vi "Interfaz grafica - corriente modf.vi"() -> ()   [LabVIEW 2024]
uses:
  TG JD - running/TG Juan Diego/Documentos de Labview/160620 Optotune Lens Driver 4 Labview package/Hello Optotune Lens (30.06.2015)/Calibration.ctl
  <vilib>/Analysis/2dsp.llb/Decimate (single shot, DBL).vi
  <vilib>/Utility/file.llb/Read Delimited Spreadsheet (string).vi
  <vilib>/Waveform/WDTOps.llb/WDT Index Channel DBL.vi
  <vilib>/Analysis/2dsp.llb/Decimate (continuous, DBL).vi
  <vilib>/Instr/_visa.llb/VISA Configure Serial Port (Instr).vi
  <vilib>/Utility/file.llb/Write Delimited Spreadsheet (string).vi
  <vilib>/Waveform/WDTOps.llb/WDT Get Waveform Time Array DBL.vi
  <vilib>/Analysis/NI_AALPro.lvlib
panel:
  in  "factor decimacion":i32=20
  in  "Parar adquisicion 2":bool
  out "Array 4":string[](array[string])
  out "Array 3":string[](array[string])
  out "Array 2":string[](array[string])
  out "Array":string[](array[string])
  out "Nombre 2":string
  in  "Restablecer Iniciales":bool
  in  "Incremento":dbl=0.1 format="%#_13g"
  out "Potencia derecho":dbl
  out "error out 4":errorcluster
  out "error out 3":errorcluster
  out "error out 2":errorcluster
  in  "Tab Control 3":enum32{"WL", "Video"}(tab)
  out "Waveform length":dbl[][](graph)
  in  "Minimo escala Y":dbl format="%#_13g"
  in  "Maximo escala Y":dbl format="%#_13g"
  in  "Escala autom. Y":u8=1
  in  "Escala autom. X":u8=1
  in  "Maximo escala X":dbl
  in  "Minimo escala X":dbl
  out "VISA resource name out":string
  in  "Tab Control 2":T1(tab)
  in  "Potencia inicial lente derecho":dbl(slide) scale=-3.0..3.0
  in  "Potencia inicial lente izquierdo":dbl(slide) scale=-3.0..3.0
  in  "VISA resource name":string="COM11"
  in  "VISA resource name 2":string="COM10"
  out "DPT INICIALES D":dbl
  out "DPT INICIALES I":dbl
  out "Potencia izquierdo":dbl
  in  "error in (no error) 5":errorcluster
  in  "error in (no error) 4":errorcluster
  in  "error in (no error) 3":errorcluster
  in  "error in (no error) 2":errorcluster
  in  "Calibration 4":T2={"Max Current A"=293.0, "Max Current B"=293.0, "UCL A"=300.0, "UCL B"=300.0, "LCL A"=0.0, "LCL B"=0.0} {"Max Current A" format="%#_g mA"; "Max Current B" format="%#_g mA"; "UCL A" format="%#_g mA"; "LCL A" format="%#_g mA"; "UCL B" format="%#_g mA"; "LCL B" format="%#_g mA"}
  out "ID 2":u16
  out "VISA resource name out 2":string
  out "Calibration 3":T2 {"Max Current A" format="%#_g mA"; "Max Current B" format="%#_g mA"; "UCL A" format="%#_g mA"; "LCL A" format="%#_g mA"; "UCL B" format="%#_g mA"; "LCL B" format="%#_g mA"}
  out "OK 2":bool
  out "Data 2":string
  out "Command to Port 2":string
  in  "Cola tipo 2":dbl[](array[numeric])
  in  "Tamaño ventana WL":i32=60
  in  "Limite inferior WL":dbl=25.0 format="%#_13g"
  in  "Limite superior WL":dbl=50.0
  out "number":u32
  in  "Calibration":T2={"Max Current A"=293.0, "Max Current B"=293.0, "UCL A"=300.0, "UCL B"=300.0, "LCL A"=0.0, "LCL B"=0.0} {"Max Current A" format="%#_g mA"; "Max Current B" format="%#_g mA"; "UCL A" format="%#_g mA"; "LCL A" format="%#_g mA"; "UCL B" format="%#_g mA"; "LCL B" format="%#_g mA"}
  out "ID":u16
  out "Calibration 2":T2 {"Max Current A" format="%#_g mA"; "Max Current B" format="%#_g mA"; "UCL A" format="%#_g mA"; "LCL A" format="%#_g mA"; "UCL B" format="%#_g mA"; "LCL B" format="%#_g mA"}
  out "OK":bool
  out "Data":string
  out "Command to Port":string
  in  "DPT dif.":dbl
  out "error out":errorcluster
  in  "error in (no error)":errorcluster
  in  "WL":dbl
  in  "Cola tipo":dbl[](array[numeric])
  out "T button?":bool
  in  "Elegir menu Exp":bool
  in  "Elegir menu":bool
  out "path":path
  in  "Iniciar experimento":bool
  in  "Parar adquisicion":bool
  out "Enfermedad visual":string
  out "Edad":string
  out "Nombre":string
  out "Cedula":string
  in  "Carpeta":path=path "C:/Users/TGM1603/Documents/LabVIEW Data/Experimentos electrodos"
  in  "?":bool
  in  "Menu Principal":u16(ring) items=["Visualizacion general ", "Llevar a cabo un experimento", "Ajustar potencia inicial lentes"]
  in  "Menu experimentos":u16(ring) items=["Experimento 1", "Experimento 2", "Experimento 3", "Experimento 4"]
  in  "Tab Control":enum32{"Señal EMG", "Potencia "}(tab)
  out "Senal EMG":waveform(dbl)[](graph)
  in  "Escala Y min":dbl
  in  "Escala Y max":dbl
  in  "Auto scale Y":u8=1
  in  "Escala X max":dbl
  in  "Escala X min":dbl
  out "Potencia Optica":dbl[](graph)
  in  "Auto scale X":u8=1
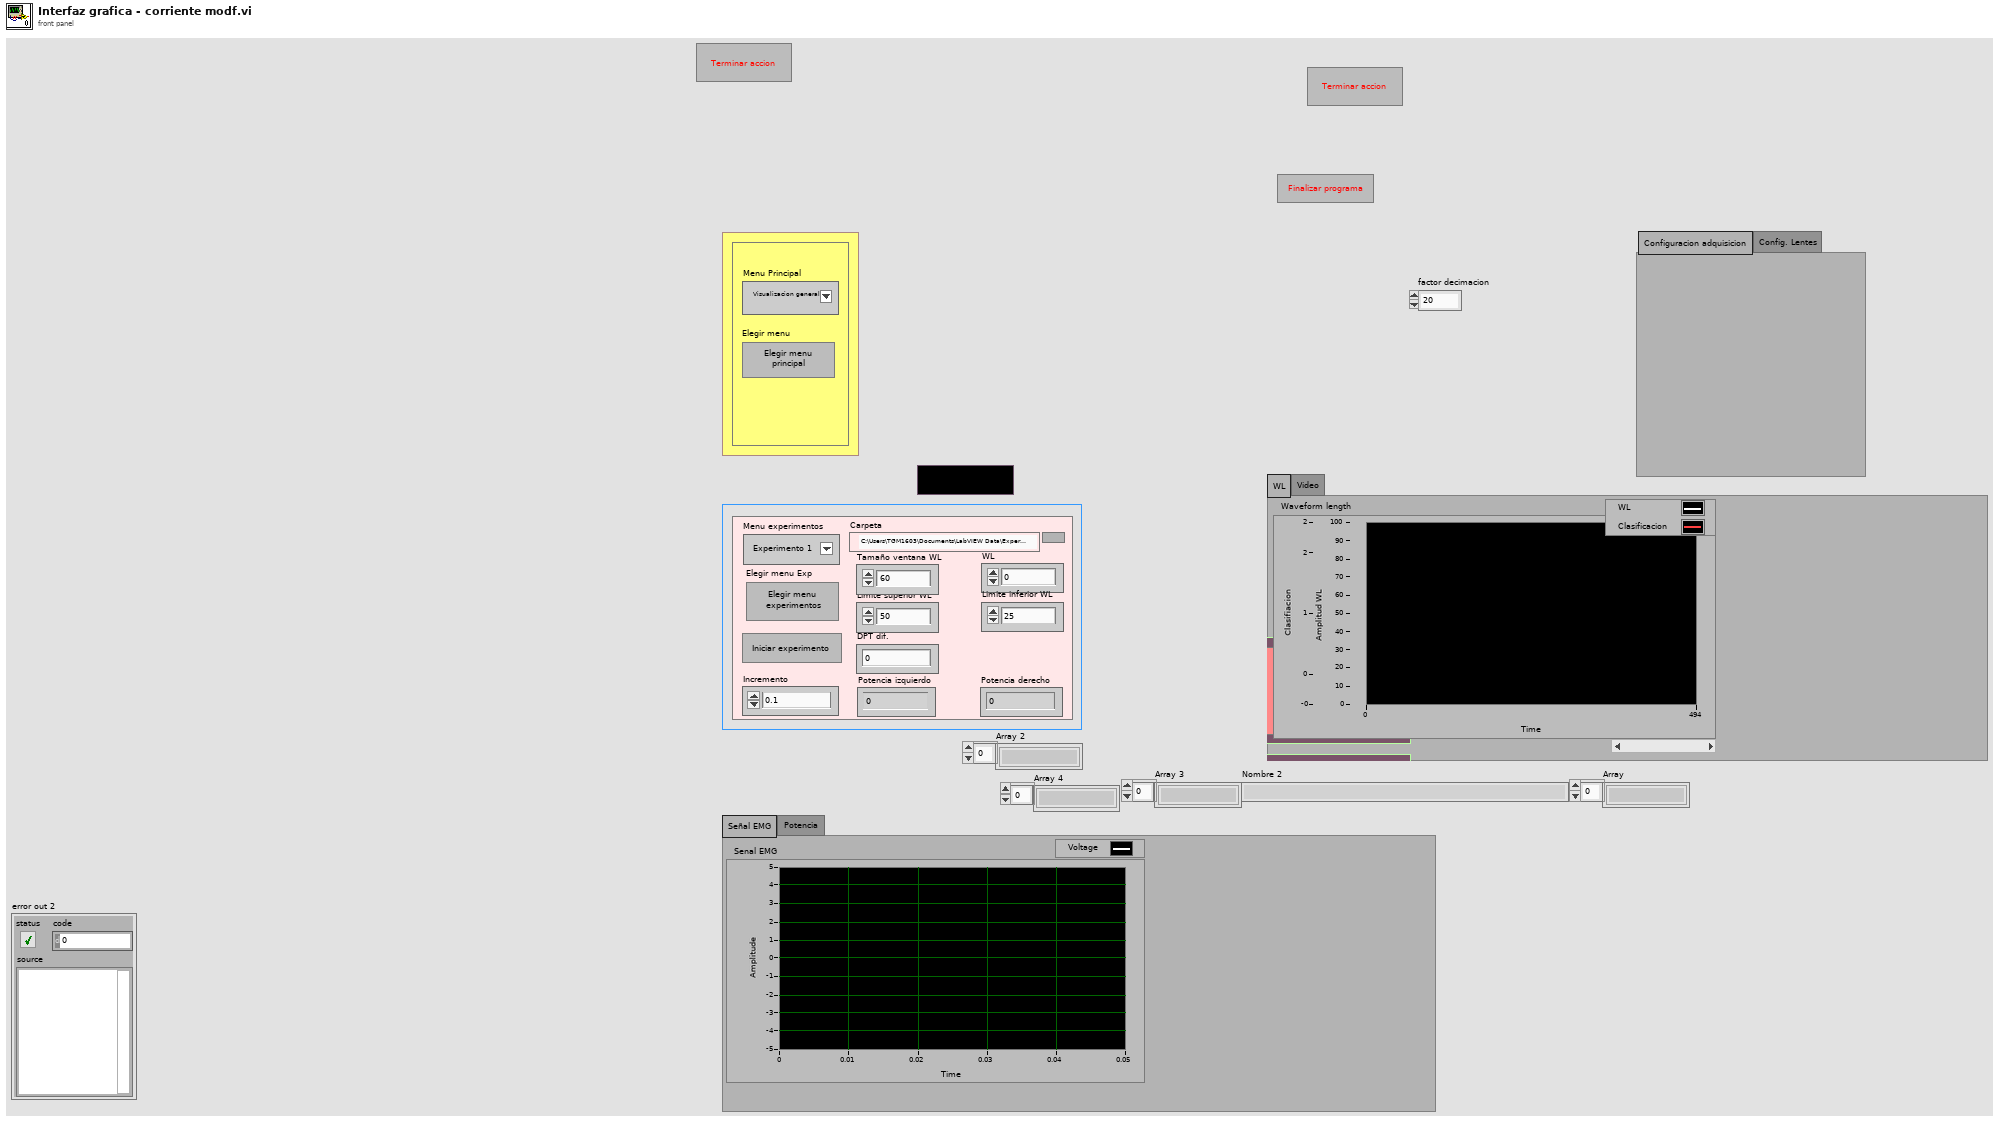
[diagram p1: front panel]
types:
  T1 = enum32{"Configuracion adquisicion", "Config. Lentes"}
  T2 = typedef "Calibration.ctl" = cluster{"Max Current A":dbl, "Max Current B":dbl, "UCL A":dbl, "UCL B":dbl, "LCL A":dbl, "LCL B":dbl}
  T3 = enum16{"Left Button", "Center Button", "Right Button", "Window Close"}
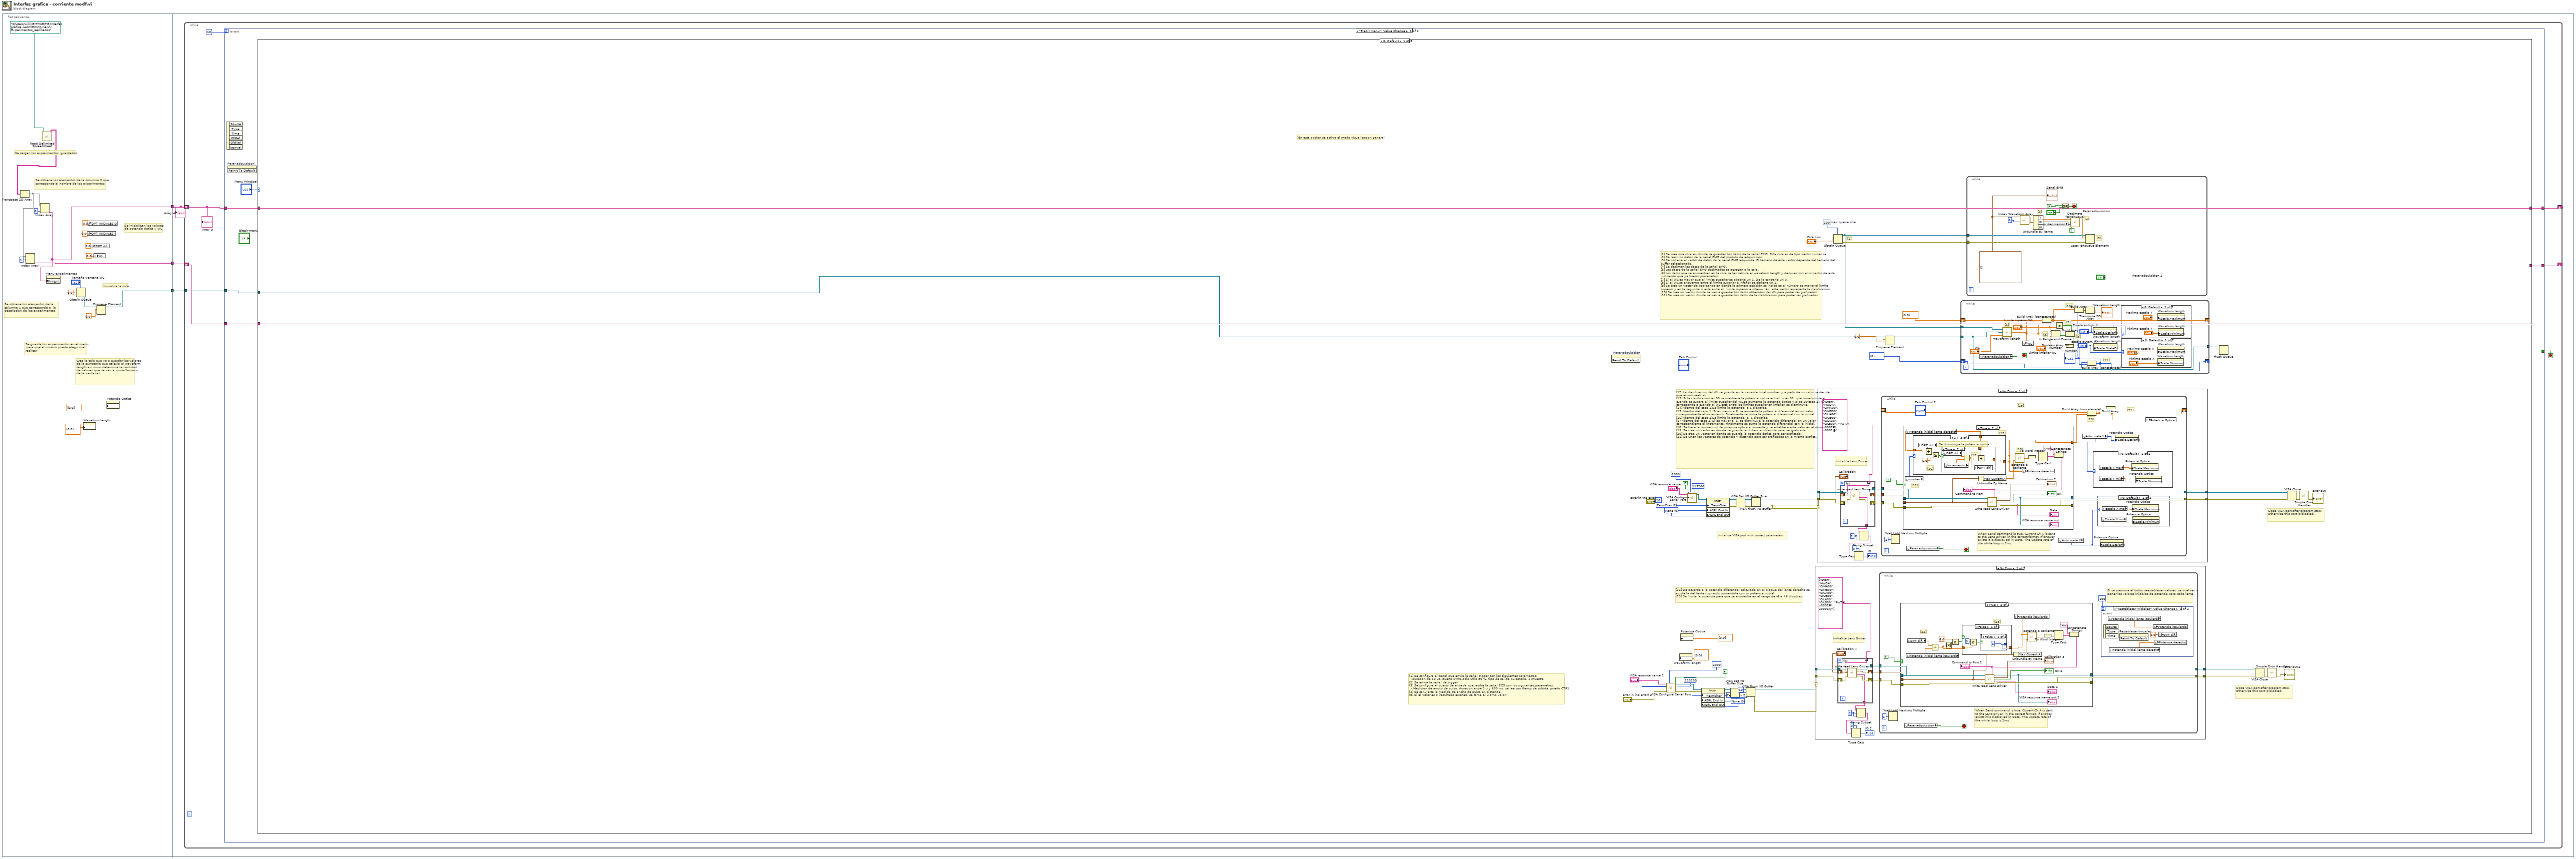
[diagram p0: block diagram]
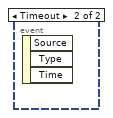
[diagram p2: hidden frame]
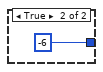
[diagram p4: hidden frame]
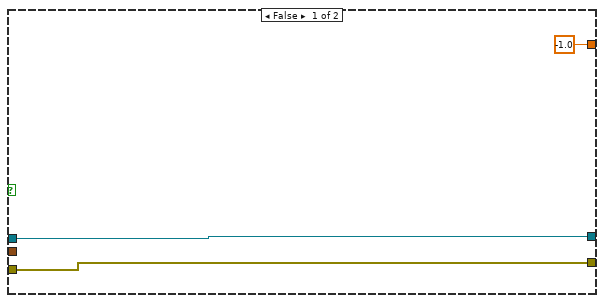
[diagram p9: hidden frame]
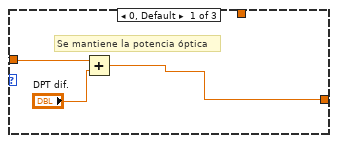
[diagram p10: hidden frame]
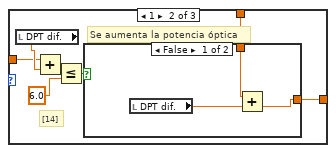
[diagram p11: hidden frame]
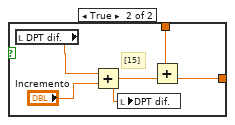
[diagram p12: hidden frame]
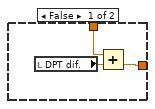
[diagram p13: hidden frame]
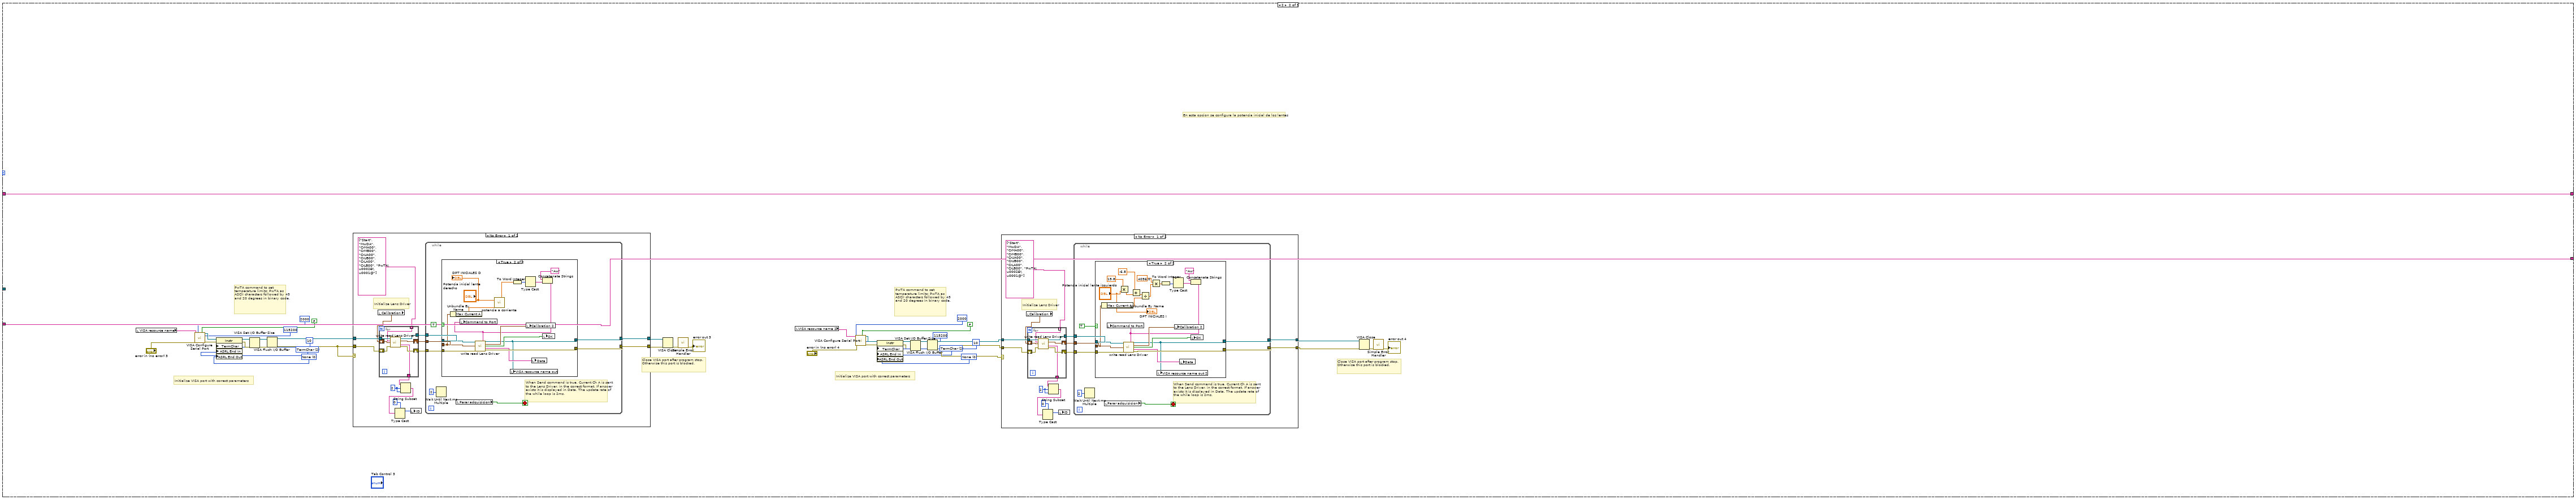
[diagram p17: hidden frame]
diagram:
  n1 = flat-sequence {
    tunnel: [w18] -> w3
    tunnel: [w15] -> w2
    tunnel: [w10] -> w1
    tunnel: w3 -> [w22]
    tunnel: w2 -> [w24]
    tunnel: w1 -> [w23]
    frame #0 {
      # "Se inicializan los valores\nde potencia óptica y WL"
      # "Inicializa la cola"
      # "Crea la cola que va a guardar los valores de la sumatoria que calcula el waveform length así como determina la cantidad de valores que se van a sumar(tamaño de la ventana)"
      # "Se obtiene los elementos de la columna 1 que corresponde a  la descripcion de los experimentos"
      # "Se obtiene los elementos de la columna 0 que corresponde al nombre de los experimentos"
      # "Se guarda los experimentos en el menu\n para que el usuario pueda elegir cual \nrealizar"
      # "Se cargan los experimentos  guardados"
      n2 = call-poly <vilib>:"Read Delimited Spreadsheet.vi"("file path (dialog if empty)"=path "C:/Users/willi/GITHUB/TG/Interfaz grafica -LabVIEW/Myne-VI/Experimentos_realizados") -> ("all rows"=w19:string[][])  [unwired: 9 in, 5 out]
      n3 = Transpose 2D Array(2D array=w19) -> (transposed array=w16:string[][])
      n4 = Index Array(array=w16, index (row)=1) -> (element=w15:string[])  [unwired: 1 in]
      n5 = Index Array(array=w16, index (row)=0) -> (element=w18:string[])  [unwired: 1 in]
      n6 = property on="Menu experimentos" class="Ring (strict)"("Strings []"=w18) -> ()  [unwired: 2 in, 2 out]
      n7 = Obtain Queue(max queue size (-1, unlimited)="Tamaño ventana WL", element data type=0.0) -> (queue out=w13:refnum<queue>)  [unwired: 3 in, 2 out]
      n8 = property on="Waveform length" class="WFChart (strict)"("History Data"=dbl[][] [[0.0]]) -> ()  [unwired: 2 in, 2 out]
      n9 = local write "DPT INICIALES D"(0.0 ("DPT INIT.1")) -> ()
      n10 = local write "DPT INICIALES I"(0.0 ("DPT INIT.2")) -> ()
      n11 = local write "DPT dif."(0.0 ("WL")) -> ()
      n12 = local write "WL"(0.0 ("WL")) -> ()
      n13 = Enqueue Element(queue=w13, element=0.0) -> (queue out=w10:refnum<queue>)  [unwired: 2 in, 2 out]
      n14 = property on="Potencia Optica" class="WFChart (strict)"("History Data"=dbl[] [0.0]) -> ()  [unwired: 2 in, 2 out]
    }
    frame #1 {
      n15 = while {
        shift-right: [w30] -> _
        shift-left: w22 -> [w31]
        shift-right: [w28] -> _
        shift-left: w24 -> [w29]
        tunnel: w23 -> [w27]
        stop <- w26 stop-if-true
        n16 = event shown="[0] \"Elegir menu\": Value Change" {
          selector: _ -> [_ _]
          dyn-events: _ -> [_ _]
          timeout: 10 -> [_ _]
          tunnel: w31 -> [w37 w914]
          tunnel: [w36 w914] -> w30
          tunnel: w29 -> [w35 w913]
          tunnel: [w34 w913] -> w28
          tunnel: w27 -> [w32 _]
          tunnel: [_ "?"] -> w26
          event "Elegir menu": Value Change {
            n17 = event-data() -> ()  [unwired: 1 in, 6 out]
            n18 = invoke on="Parar adquisicion" class="Bool (strict)" method="Reinit To Default"() -> ()  [unwired: 3 in, 3 out]
            n19 = case shown="0, Default" "Menu Principal" {
              tunnel: w37 -> [w91 w328 w448]
              tunnel: [w91 w328 w447] -> w36
              tunnel: w35 -> [w90 w327 w445]
              tunnel: [w90 w327 w444] -> w34
              tunnel: w32 -> [w85 _ w435]
              frame 0, Default {
                w53 = u16 0 items=["None", "Last Bit", "TermChar", "Break"] ("Serial Settings:End Mode for Writes")
                w52 = u16 2 items=["None", "Last Bit", "TermChar"] ("Serial Settings:End Mode for Reads")
                w75 = u16 0 items=["None", "Last Bit", "TermChar", "Break"] ("Serial Settings:End Mode for Writes")
                w76 = u16 2 items=["None", "Last Bit", "TermChar"] ("Serial Settings:End Mode for Reads")
                w89 = 100  # max queue size
                # "[22] De acuerda a la potencia diferencial calculada en el bloque del lente derecho se ajusta la del lente izquierdo sumandola con su potencia inicial.\n[23] Se limita la potencia para que se encuentre en el rango de -6 a +6 dioptrías."
                # "[12] La clasificación del WL se guarda en la variable local number, y a partir de su valor se decide que accion realizar.\n[13] Si la clasificacion es 00 se mantiene la potencia óptica actual, si es 01, que corresponde a cuando se supera el limite superior del WL,se aumenta la potencia óptica y si es 10(caso 2), que corresponde a cuando el WL está entre los limites superior en inferior, se disminuye. \n[14] (dentro del caso 1)Se limita la potencia  a 6 dioptrías. \n[15] (dentro del caso 1) Si es menor a 6, se aumenta la potencia diferencial en un valor correspondiente al incremento. Finalmente se suma la potencia diferencial con la inicial.\n[16] (dentro del caso 2)Se limita la potencia  a -6 dioptrías.\n[17 (dentro del caso 2) Si es mayor a -6, se disminuye la potencia diferencial en un valor correspondiente al incremento. Finalmente se suma la potencia diferencial con la inicial.\n[18] Se hace la conversión de potencia óptica a corriente y se establece este valor en el driver.\n[19] Se crea un vector en donde se guarda la distancia obtenida para ser graficada.\n[20] Se crea un vector en donde se guarda la potencia óptica para ser graficada.\n[21] Se unen los vectores de potencia y distancia para ser graficados en la misma grafica."
                # "[1] Se crea una cola en donde se guardan los datos de la señal EMG. Esta cola es de tipo vector numerica.\n[2] Se leen los datos de la señal EMG del módulo de adquisición. \n[3] Se obtiene el vector de datos de la señal EMG adquirida. El tamaño de este vector depende del tamaño del buffer seleccionado.\n[4] Se deciman los datos de la señal EMG.\n[5] Los datos de la señal EMG decimados se agregan a la cola.\n[6] Los datos que se encuentran en la cola se les calcula el waveform length y después son eliminados de esta, indicando que ya fueron procesados. \n[7] Si el WL es mayor que el limite superior se obtiene un 1. De lo contrario un 0.\n[8] Si el WL se encuentra entre el límite superior e infefior se obtiene un 1.\n[9] Se crea un vector de booleanos en donde la primera posición se indica se el número es mayor al límite superior y en la segunda si está entre el  limite superior e inferior. Así, este vector representa la clasificación.\n[10] Se crea un vector donde se van a guardar los datos obtenidos del WL para poder ser graficados.\n[11] Se crea un vector donde se van a guardar los datos de la clasificación para poder ser graficados."
                # "[1]"
                # "En esta opcion se activa el modo visualizacion general"
                # "Close VISA port after program stop. Otherwise this port is blocked."
                # "[1] Se configura el canal que envía la señal trigger con los siguientes parametros:\n  -duracion de 10 us, puerto CTR0,ciclo utilo 50 %, tipo de salida pulsatoria, 1 muestra \n[2] Se envía la señal de trigger.\n[3] Se configura el puerto de entrada que recibe la señal ECO con los siguientes parámetros:\n  - Medicion de ancho de pulso, duracion entre 1 u y 600 ms, se lee con flanco de subida, puerto CTR1\n[4] Se convierte la medida de ancho de pulso en distancia.\n[5] Si el valor es 0 (resultado erroneo) se toma el último valor."
                # "Close VISA port after program stop. Otherwise this port is blocked."
                # "Initialize VISA port with correct parameters"
                n20 = invoke on="Parar adquisicion" class="Bool (strict)" method="Reinit To Default"() -> ()  [unwired: 3 in, 3 out]
                n21 = call-poly "VISA Configure Serial Port"("VISA resource name"="VISA resource name 2", "timeout (10sec)"=u32 2000, "Enable Termination\nChar (T)"=FALSE ("Enable Termination\nChar (T)"), "baud rate (9600)"=u32 115200, "error in (no error)"="error in (no error) 2") -> ("VISA resource name out"=w48:refnum<visa-resource-name>, "error out"=w50:errorcluster)  [unwired: 9 in]
                n22 = property on="Waveform length" class="WFChart (strict)"("History Data"=dbl[][] [[0.0]]) -> ()  [unwired: 2 in, 2 out]
                n23 = property on="Potencia Optica" class="WFChart (strict)"("History Data"=dbl[] [0.0]) -> ()  [unwired: 2 in, 2 out]
                n24 = call-poly "VISA Configure Serial Port"("VISA resource name"="VISA resource name", "timeout (10sec)"=u32 2000, "Enable Termination\nChar (T)"=FALSE ("Enable Termination\nChar (T)"), "baud rate (9600)"=u32 115200, "error in (no error)"="error in (no error)") -> ("VISA resource name out"=w80:refnum<visa-resource-name>, "error out"=w78:errorcluster)  [unwired: 9 in]
                n25 = property class="Instr"(reference=w48, error in=w50, "TermChar"=u8 10 ("Message Based Settings:Termination Character"), "ASRL End In"=w52, "ASRL End Out"=w53) -> (reference out=w49:refnum<visa-resource-name>, error out=w51:errorcluster)
                n26 = property class="Instr"(reference=w80, error in=w78, "TermChar"=u8 10 ("Message Based Settings:Termination Character"), "ASRL End In"=w76, "ASRL End Out"=w75) -> (reference out=w79:refnum<visa-resource-name>, error out=w77:errorcluster)
                n27 = VISA Set I/O Buffer Size(VISA resource name=w49, error in (no error)=w51) -> (VISA resource name out=w56:refnum<visa-resource-name>, error out=w57:errorcluster)  [unwired: 2 in]
                n28 = VISA Set I/O Buffer Size(VISA resource name=w79, error in (no error)=w77) -> (VISA resource name out=w72:refnum<visa-resource-name>, error out=w71:errorcluster)  [unwired: 2 in]
                n29 = VISA Flush I/O Buffer(VISA resource name=w56, error in (no error)=w57) -> (VISA resource name out=w42:refnum<visa-resource-name>, error out=w43:errorcluster)  [unwired: 1 in]
                n30 = VISA Flush I/O Buffer(VISA resource name=w72, error in (no error)=w71) -> (VISA resource name out=w70:refnum<visa-resource-name>, error out=w65:errorcluster)  [unwired: 1 in]
                n31 = case shown="No Error" w43 {
                  tunnel: w43 -> [w105 w156]
                  tunnel: w42 -> [w104 w157]
                  tunnel: [w103 w156] -> w38
                  tunnel: [w102 w157] -> w39
                  frame No Error {
                    w100 = 2 ("length (rest)")
                    # "Initialize Lens Driver"
                    n32 = for {
                      tunnel: w104 -> [w154]
                      tunnel: [w151] -> w94
                      tunnel: string[] ["Start", "MwDA", "CrMA00", "CrMB00", "CrUA00", "CrUB00", "CrLA00", "CrLB00", "PwTA\u0002Ð\u0001@"] -> [w149] mode=indexing
                      tunnel: [w148] -> w93
                      shift-right: [w152] -> w95
                      shift-left: "Calibration 4" -> [w153]
                      shift-right: [w150] -> w96
                      shift-left: w105 -> [w155]
                      n33 = call "write read Lens Driver.vi"("VISA resource name"=w154, "command"=w149, "Calibration"=w153, "error in (no error)"=w155) -> ("VISA resource name out"=w151:refnum<visa-resource-name>, "Calibration 2"=w152:T2, "Data"=w148:string, "error out"=w150:errorcluster)  [unwired: 4 in, 4 out]
                    }
                    n34 = String Subset(string=w93, offset (0)=w100, length (rest)=w100) -> (substring=w98:string)
                    n35 = Type Cast(type=u16 0 ("length (rest)"), x=w98) -> (*(type *) &x=→"ID 2":u16)
                    n36 = while {
                      tunnel: [w108] -> w103
                      tunnel: [w109] -> w102
                      tunnel: w96 -> [w114]
                      tunnel: w95 -> [w113]
                      tunnel: w94 -> [w112]
                      stop <- w107 stop-if-true
                      # "Si se presiona el botón reestablecer valores, se vuelven a poner los valores iniciales de potencia para cada lente"
                      # "When Send command is true, Current Ch A is sent to the Lens Driver, in the correct format. If answer exists it is displayed in Data. The update rate of the while loop is 2ms."
                      n37 = Wait Until Next ms Multiple(millisecond multiple=u32 2) -> ()  [unwired: 1 out]
                      n38 = case shown="True" TRUE ("Send command") {
                        tunnel: [w119 w140] -> w108
                        tunnel: w114 -> [w119 w139]
                        tunnel: w113 -> [_ w121]
                        tunnel: w112 -> [w118 w138]
                        tunnel: [w118 w135] -> w109
                        frame False {
                        }
                        frame True {
                          # "[23]"
                          # "[22]"
                          n39 = local read "Potencia inicial lente izquierdo"() -> (w129:dbl)
                          n40 = local read "DPT dif."() -> (w130:dbl)
                          n41 = Add(x=w130, y=w129) -> (x+y=w125:dbl)
                          n42 = Absolute Value(x=w125) -> (abs(x)=w127:dbl)
                          n43 = Greater Or Equal?(x=6.0, y=w127) -> (x >= y?=w128:bool)
                          n44 = case shown="False" w128 {
                            tunnel: w125 -> [w143 w147]
                            tunnel: [w141 w147] -> w123
                            frame False {
                              n45 = Greater Or Equal?(x=u16 0, y=w143) -> (x >= y?=w144:bool)
                              n46 = case shown="False" w144 {
                                tunnel: [i16 6 ("x") i16 -6 ("x")] -> w141
                                frame False {
                                }
                                frame True {
                                }
                              }
                            }
                            frame True {
                            }
                          }
                          n47 = Unbundle By Name(w121) -> ("Max Current A"=w122:dbl)
                          n48 = local write "Potencia izquierdo"(w123) -> ()
                          n49 = call "potencia a corriente.vi"("Max current A"=w122, "Potencia"=w123) -> ("Corriente"=w124:dbl)
                          n50 = To Word Integer(number=w124) -> (16bit integer=w133:i16)
                          n51 = Type Cast(x=w133) -> (*(type *) &x=w132:string)  [unwired: 1 in]
                          n52 = Concatenate Strings("Aw", w132) -> (w131:string)
                          "Command to Port 2" <- w131
                          n53 = call "write read Lens Driver.vi"("VISA resource name"=w138, "command"=w131, "Calibration"=w121, "error in (no error)"=w139) -> ("VISA resource name out"=w135:refnum<visa-resource-name>, "Calibration 2"=→"Calibration 3":T2, "OK"=→"OK 2":bool, "Data"=→"Data 2":string, "error out"=w140:errorcluster)  [unwired: 4 in, 3 out]
                          "VISA resource name out 2" <- w135
                        }
                      }
                      n54 = local read "Parar adquisicion"() -> (w107:bool)
                      n55 = event shown="[0] \"Restablecer Iniciales\": Value Change" {
                        selector: _ -> [_ _]
                        dyn-events: _ -> [_ _]
                        timeout: 100 -> [_ _]
                        event "Restablecer Iniciales": Value Change {
                          n56 = event-data() -> ()  [unwired: 1 in, 3 out]
                          n57 = local read "Potencia inicial lente izquierdo"() -> (w115:dbl)
                          n58 = local read "Potencia inicial lente derecho"() -> (w116:dbl)
                          n59 = invoke on="Restablecer Iniciales" class="Bool" method="Reinit To Default"() -> ()  [unwired: 3 in, 3 out]
                          n60 = local write "Potencia izquierdo"(w115) -> ()
                          n61 = local write "Potencia derecho"(w116) -> ()
                          n62 = local write "DPT dif."(0.0 ("DPT dif.")) -> ()
                        }
                        event Timeout {
                          n63 = event-data() -> ()  [unwired: 1 in, 3 out]
                        }
                      }
                    }
                  }
                  frame Error {
                  }
                }
                n64 = case shown="No Error" w65 {
                  tunnel: w65 -> [w171 w250]
                  tunnel: w70 -> [w170 w251]
                  tunnel: [w169 w250] -> w68
                  tunnel: [w168 w251] -> w66
                  frame No Error {
                    w166 = 2 ("length (rest)")
                    # "Initialize Lens Driver"
                    n65 = for {
                      tunnel: w170 -> [w248]
                      tunnel: [w245] -> w160
                      tunnel: string[] ["Start", "MwDA", "CrMA00", "CrMB00", "CrUA00", "CrUB00", "CrLA00", "CrLB00", "PwTA\u0002Ð\u0001@"] -> [w243] mode=indexing
                      tunnel: [w242] -> w159
                      shift-right: [w246] -> w161
                      shift-left: "Calibration" -> [w247]
                      shift-right: [w244] -> w162
                      shift-left: w171 -> [w249]
                      n66 = call "write read Lens Driver.vi"("VISA resource name"=w248, "command"=w243, "Calibration"=w247, "error in (no error)"=w249) -> ("VISA resource name out"=w245:refnum<visa-resource-name>, "Calibration 2"=w246:T2, "Data"=w242:string, "error out"=w244:errorcluster)  [unwired: 4 in, 4 out]
                    }
                    n67 = String Subset(string=w159, offset (0)=w166, length (rest)=w166) -> (substring=w164:string)
                    n68 = Type Cast(type=u16 0 ("length (rest)"), x=w164) -> (*(type *) &x=→"ID":u16)
                    n69 = while {
                      tunnel: [w178] -> w169
                      tunnel: [w179] -> w168
                      tunnel: w162 -> [w184]
                      tunnel: w161 -> [w183]
                      tunnel: w160 -> [w182]
                      shift-right: [w172] -> _
                      shift-left: _ -> [w174]
                      stop <- w177 stop-if-true
                      # "[21]"
                      # "[20]"
                      # "[19]"
                      # "When Send command is true, Current Ch A is sent to the Lens Driver, in the correct format. If answer exists it is displayed in Data. The update rate of the while loop is 2ms."
                      n70 = Wait Until Next ms Multiple(millisecond multiple=u32 2) -> ()  [unwired: 1 out]
                      n71 = case shown="True" TRUE ("Send command") {
                        tunnel: [w191 w208] -> w178
                        tunnel: w184 -> [w191 w207]
                        tunnel: w183 -> [_ w194]
                        tunnel: w182 -> [w190 w206]
                        tunnel: [w190 w203] -> w179
                        tunnel: [-1.0 ("DPT") w196] -> w173
                        frame False {
                        }
                        frame True {
                          # "[18]"
                          # "[13]"
                          # "[12]"
                          n72 = local read "number"() -> (w198:u32)
                          n73 = local read "Potencia inicial lente derecho"() -> (w197:dbl)
                          n74 = case shown="2" w198 {
                            tunnel: [w210 w218 w233] -> w196
                            tunnel: w197 -> [w211 w213 w228]
                            tunnel: w197 -> [_ w212 w227]
                            frame 0, Default {
                              # "Se mantiene la potencia óptica"
                              n75 = Add(x=w211, y="DPT dif.") -> (x+y=w210:dbl)
                            }
                            frame 1 {
                              # "[14]"
                              # "Se aumenta la potencia óptica"
                              n76 = local read "DPT dif."() -> (w214:dbl)
                              n77 = Add(x=w213, y=w214) -> (x+y=w215:dbl)
                              n78 = Less Or Equal?(x=w215, y=6.0) -> (x <= y?=w217:bool)
                              n79 = case shown="False" w217 {
                                tunnel: [w220 w223] -> w218
                                tunnel: w212 -> [w219 w222]
                                frame False {
                                n80 = local read "DPT dif."() -> (w221:dbl)
                                n81 = Add(x=w219, y=w221) -> (x+y=w220:dbl)
                                }
                                frame True {
                                # "[15]"
                                n82 = local read "DPT dif."() -> (w224:dbl)
                                n83 = Add(x=w224, y="Incremento") -> (x+y=w225:dbl)
                                n84 = local write "DPT dif."(w225) -> ()
                                n85 = Add(x=w222, y=w225) -> (x+y=w223:dbl)
                                }
                              }
                            }
                            frame 2 {
                              # "[16]"
                              # "Se disminuye la potencia óptica"
                              n86 = local read "DPT dif."() -> (w232:dbl)
                              n87 = Add(x=w232, y=w228) -> (x+y=w229:dbl)
                              n88 = Greater Or Equal?(x=w229, y=-6.0) -> (x >= y?=w230:bool)
                              n89 = case shown="True" w230 {
                                tunnel: [w235 w239] -> w233
                                tunnel: w227 -> [w234 w238]
                                frame False {
                                n90 = local read "DPT dif."() -> (w236:dbl)
                                n91 = Add(x=w234, y=w236) -> (x+y=w235:dbl)
                                }
                                frame True {
                                # "[17]"
                                n92 = local read "DPT dif."() -> (w241:dbl)
                                n93 = local read "Incremento"() -> (w237:dbl)
                                n94 = Subtract(x=w241, y=w237) -> (x-y=w240:dbl)
                                n95 = local write "DPT dif."(w240) -> ()
                                n96 = Add(x=w238, y=w240) -> (x+y=w239:dbl)
                                }
                              }
                            }
                          }
                          n97 = Unbundle By Name(w194) -> ("Max Current A"=w193:dbl)
                          n98 = call "potencia a corriente.vi"("Max current A"=w193, "Potencia"=w196) -> ("Corriente"=w195:dbl)
                          n99 = local write "Potencia derecho"(w196) -> ()
                          n100 = To Word Integer(number=w195) -> (16bit integer=w201:i16)
                          n101 = Type Cast(x=w201) -> (*(type *) &x=w200:string)  [unwired: 1 in]
                          n102 = Concatenate Strings("Aw", w200) -> (w199:string)
                          "Command to Port" <- w199
                          n103 = call "write read Lens Driver.vi"("VISA resource name"=w206, "command"=w199, "Calibration"=w194, "error in (no error)"=w207) -> ("VISA resource name out"=w203:refnum<visa-resource-name>, "Calibration 2"=→"Calibration 2":T2, "OK"=→"OK":bool, "Data"=→"Data":string, "error out"=w208:errorcluster)  [unwired: 4 in, 3 out]
                          "VISA resource name out" <- w203
                        }
                      }
                      n104 = local read "Parar adquisicion"() -> (w177:bool)
                      n105 = local read "Auto scale X"() -> (w175:u8)
                      n106 = local read "Auto scale Y"() -> (w176:u8)
                      n107 = Build Array (concatenate)(w174, w173) -> (w172:dbl[])
                      n108 = case shown="0, Default" w176 {
                        frame 0, Default {
                          n109 = local read "Escala Y max"() -> (w188:dbl)
                          n110 = local read "Escala Y min"() -> (w187:dbl)
                          n111 = property on="Potencia Optica" class="WFChart (strict)"("YScale.Maximum"=w188) -> ()  [unwired: 2 in, 2 out]
                          n112 = property on="Potencia Optica" class="WFChart (strict)"("YScale.Minimum"=w187) -> ()  [unwired: 2 in, 2 out]
                        }
                        frame 1 {
                        }
                      }
                      n113 = case shown="0, Default" w175 {
                        frame 0, Default {
                          n114 = local read "Escala X min"() -> (w185:dbl)
                          n115 = local read "Escala X max"() -> (w186:dbl)
                          n116 = property on="Potencia Optica" class="WFChart (strict)"("XScale.Maximum"=w186) -> ()  [unwired: 2 in, 2 out]
                          n117 = property on="Potencia Optica" class="WFChart (strict)"("XScale.Minimum"=w185) -> ()  [unwired: 2 in, 2 out]
                        }
                        frame 1 {
                        }
                      }
                      n118 = property on="Potencia Optica" class="WFChart (strict)"("XScale.ScaleFit"=w175) -> ()  [unwired: 2 in, 2 out]
                      n119 = Build Array(w172) -> ()  [unwired: 1 out]
                      n120 = property on="Potencia Optica" class="WFChart (strict)"("YScale.ScaleFit"=w176) -> ()  [unwired: 2 in, 2 out]
                      n121 = local write "Potencia Optica"(w172) -> ()
                    }
                  }
                  frame Error {
                  }
                }
                n122 = Obtain Queue(max queue size (-1, unlimited)=w89, element data type="Cola tipo") -> (queue out=w86:refnum<queue>, error out=w87:errorcluster)  [unwired: 3 in, 1 out]
                n123 = Enqueue Element(queue=w85, element=0.0) -> (queue out=w62:refnum<queue>)  [unwired: 2 in, 2 out]
                n124 = while {
                  tunnel: w62 -> [w253]
                  tunnel: w86 -> [w270]
                  shift-right: [w256] -> _
                  shift-left: dbl[] [0.0] -> [w267]
                  shift-right: [w255] -> _
                  shift-left: u32[] [0] -> [w257]
                  tunnel: [w253] -> w60
                  stop <- w268 stop-if-true
                  # "[11]"
                  # "[10]"
                  # "[9]"
                  # "[8]"
                  # "[7]"
                  # "[6]"
                  n125 = local read "Parar adquisicion"() -> (w268:bool)
                  n126 = call "waveform_length.vi"("WL"="WL", "Cola WL"=w253, "Datos entrada"=w270) -> ("WL 2"=w265:dbl)
                  n127 = local write "WL"(w265) -> ()
                  n128 = Build Array (concatenate)(w267, w265) -> (w256:dbl[])
                  n129 = In Range and Coerce(upper limit="Limite superior WL", x=w265, lower limit="Limite inferior WL") -> (In Range?=w263:bool)  [unwired: 1 out]
                  n130 = Greater?(x=w265, y="Limite superior WL") -> (0:w264:bool)
                  n131 = Build Array(w264, w263) -> (w262:bool[])
                  n132 = Boolean Array To Number(Boolean array=w262) -> (number=w258:u32)
                  "number" <- w258
                  n133 = Build Array (concatenate)(w257, w258) -> (w255:u32[])
                  n134 = Build Array(w256, w255) -> (w254:dbl[][])
                  n135 = Transpose 2D Array(2D array=w254) -> (transposed array=→"Waveform length":dbl[][])
                  n136 = property on="Waveform length" class="WFChart (strict)"("YScale.ScaleFit"="Escala autom. Y") -> ()  [unwired: 2 in, 2 out]
                  n137 = property on="Waveform length" class="WFChart (strict)"("XScale.ScaleFit"="Escala autom. X") -> ()  [unwired: 2 in, 2 out]
                  n138 = case shown="0, Default" "Escala autom. Y" {
                    frame 0, Default {
                      n139 = property on="Waveform length" class="WFChart (strict)"("YScale.Maximum"="Maximo escala Y") -> ()  [unwired: 2 in, 2 out]
                      n140 = property on="Waveform length" class="WFChart (strict)"("YScale.Minimum"="Minimo escala Y") -> ()  [unwired: 2 in, 2 out]
                    }
                    frame 1 {
                    }
                  }
                  n141 = case shown="0, Default" "Escala autom. X" {
                    frame 0, Default {
                      n142 = property on="Waveform length" class="WFChart (strict)"("XScale.Minimum"="Minimo escala X") -> ()  [unwired: 2 in, 2 out]
                      n143 = property on="Waveform length" class="WFChart (strict)"("XScale.Maximum"="Maximo escala X") -> ()  [unwired: 2 in, 2 out]
                    }
                    frame 1 {
                    }
                  }
                }
                n144 = while {
                  tunnel: w86 -> [w279]
                  tunnel: w87 -> [w278]
                  stop <- w286 stop-if-true
                  w276 = waveform(dbl)[] [] ("waveform array")
                  # "[5]"
                  # "[4]"
                  # "[3]"
                  n145 = call-poly <vilib>:"Index Waveform Array.vi"("index"=0, "waveform array"=w276) -> ("waveform"=w283:waveform(dbl))  [unwired: 8 in, 1 out]
                  n146 = Unbundle By Name(w283) -> ("Y"=w281:dbl[])  [unwired: 2 out]
                  n147 = local read "factor decimacion"() -> (w280:i32)
                  n148 = Or(x=FALSE, y="Parar adquisicion") -> (x .or. y?=w286:bool)
                  n149 = call-poly <vilib>:"Decimate (continuous).vi"("averaging"=TRUE, "decimating factor"=w280, "X"=w281) -> ("Decimated Array"=w277:dbl[])  [unwired: 7 in, 1 out]
                  n150 = Lossy Enqueue Element(queue=w279, element=w277, error in (no error)=w278) -> ()  [unwired: 4 out]
                  "Senal EMG" <- w276
                }
                n151 = Flush Queue(queue=w60) -> ()  [unwired: 1 in, 3 out]
                n152 = VISA Close(VISA resource name=w39, error in (no error)=w38) -> (error out=w40:errorcluster)
                n153 = call <vilib>:"Simple Error Handler.vi"("error in (no error)"=w40) -> ("error out"=→"error out 2":errorcluster)  [unwired: 4 in, 4 out]
                n154 = VISA Close(VISA resource name=w66, error in (no error)=w68) -> (error out=w69:errorcluster)
                n155 = call <vilib>:"Simple Error Handler.vi"("error in (no error)"=w69) -> ("error out"=→"error out":errorcluster)  [unwired: 4 in, 4 out]
              }
              frame 2 {
                w307 = u16 0 items=["None", "Last Bit", "TermChar", "Break"] ("Serial Settings:End Mode for Writes")
                w306 = u16 2 items=["None", "Last Bit", "TermChar"] ("Serial Settings:End Mode for Reads")
                w320 = u16 0 items=["None", "Last Bit", "TermChar", "Break"] ("Serial Settings:End Mode for Writes")
                w319 = u16 2 items=["None", "Last Bit", "TermChar"] ("Serial Settings:End Mode for Reads")
                # "En esta opcion se configura la potencia inicial de los lentes"
                # "Close VISA port after program stop. Otherwise this port is blocked."
                # "Close VISA port after program stop. Otherwise this port is blocked."
                # "PwTA command to set temperature limits: PwTA as ASCII characters followed by 45 and 20 degrees in binary code."
                # "Initialize VISA port with correct parameters"
                # "PwTA command to set temperature limits: PwTA as ASCII characters followed by 45 and 20 degrees in binary code."
                # "Initialize VISA port with correct parameters"
                n156 = local read "VISA resource name"() -> (w297:string)
                n157 = call-poly "VISA Configure Serial Port"("VISA resource name"=w297, "timeout (10sec)"=u32 2000, "Enable Termination\nChar (T)"=FALSE ("Enable Termination\nChar (T)"), "baud rate (9600)"=u32 115200, "error in (no error)"="error in (no error) 3") -> ("VISA resource name out"=w302:refnum<visa-resource-name>, "error out"=w304:errorcluster)  [unwired: 9 in]
                n158 = property class="Instr"(reference=w302, error in=w304, "TermChar"=u8 10 ("Message Based Settings:Termination Character"), "ASRL End In"=w306, "ASRL End Out"=w307) -> (reference out=w303:refnum<visa-resource-name>, error out=w305:errorcluster)
                n159 = VISA Set I/O Buffer Size(VISA resource name=w303, error in (no error)=w305) -> (VISA resource name out=w309:refnum<visa-resource-name>, error out=w310:errorcluster)  [unwired: 2 in]
                n160 = VISA Flush I/O Buffer(VISA resource name=w309, error in (no error)=w310) -> (VISA resource name out=w296:refnum<visa-resource-name>, error out=w295:errorcluster)  [unwired: 1 in]
                n161 = case shown="No Error" w295 {
                  tunnel: w295 -> [w342 w376]
                  tunnel: w296 -> [w341 w377]
                  tunnel: [w340 w376] -> w291
                  tunnel: [w339 w377] -> w292
                  frame No Error {
                    w338 = 2 ("length (rest)")
                    # "Initialize Lens Driver"
                    n162 = local read "Calibration"() -> (w330:T2)
                    n163 = for {
                      tunnel: w341 -> [w374]
                      tunnel: [w371] -> w333
                      tunnel: string[] ["Start", "MwDA", "CrMA00", "CrMB00", "CrUA00", "CrUB00", "CrLA00", "CrLB00", "PwTA\u0002Ð\u0001@"] -> [w369] mode=indexing
                      tunnel: [w368] -> w332
                      shift-right: [w372] -> w334
                      shift-left: w330 -> [w373]
                      shift-right: [w370] -> w335
                      shift-left: w342 -> [w375]
                      n164 = call "write read Lens Driver.vi"("VISA resource name"=w374, "command"=w369, "Calibration"=w373, "error in (no error)"=w375) -> ("VISA resource name out"=w371:refnum<visa-resource-name>, "Calibration 2"=w372:T2, "Data"=w368:string, "error out"=w370:errorcluster)  [unwired: 4 in, 4 out]
                    }
                    n165 = String Subset(string=w332, offset (0)=w338, length (rest)=w338) -> (substring=w336:string)
                    n166 = Type Cast(type=u16 0 ("length (rest)"), x=w336) -> (*(type *) &x=w331:u16)
                    n167 = local write "ID"(w331) -> ()
                    n168 = while {
                      tunnel: [w344] -> w340
                      tunnel: [w345] -> w339
                      tunnel: w335 -> [w350]
                      tunnel: w334 -> [w349]
                      tunnel: w333 -> [w348]
                      stop <- w343 stop-if-true
                      # "When Send command is true, Current Ch A is sent to the Lens Driver, in the correct format. If answer exists it is displayed in Data. The update rate of the while loop is 2ms."
                      n169 = Wait Until Next ms Multiple(millisecond multiple=u32 2) -> ()  [unwired: 1 out]
                      n170 = case shown="True" TRUE ("Send command") {
                        tunnel: [w352 w367] -> w344
                        tunnel: w350 -> [w352 w366]
                        tunnel: w349 -> [_ w357]
                        tunnel: w348 -> [w351 w365]
                        tunnel: [w351 w358] -> w345
                        frame False {
                        }
                        frame True {
                          n171 = Unbundle By Name(w357) -> ("Max Current A"=w356:dbl)
                          n172 = call "potencia a corriente.vi"("Max current A"=w356, "Potencia"="Potencia inicial lente derecho") -> ("Corriente"=w354:dbl)
                          n173 = To Word Integer(number=w354) -> (16bit integer=w364:i16)
                          n174 = Type Cast(x=w364) -> (*(type *) &x=w363:string)  [unwired: 1 in]
                          n175 = Concatenate Strings("Aw", w363) -> (w360:string)
                          n176 = local write "Command to Port"(w360) -> ()
                          n177 = call "write read Lens Driver.vi"("VISA resource name"=w365, "command"=w360, "Calibration"=w357, "error in (no error)"=w366) -> ("VISA resource name out"=w358:refnum<visa-resource-name>, "Calibration 2"=w362:T2, "OK"=w361:bool, "Data"=w359:string, "error out"=w367:errorcluster)  [unwired: 4 in, 3 out]
                          n178 = local write "VISA resource name out"(w358) -> ()
                          n179 = local write "Calibration 2"(w362) -> ()
                          n180 = local write "Data"(w359) -> ()
                          n181 = local write "OK"(w361) -> ()
                          "DPT INICIALES D" <- "Potencia inicial lente derecho"
                        }
                      }
                      n182 = local read "Parar adquisicion"() -> (w343:bool)
                    }
                  }
                  frame Error {
                  }
                }
                n183 = VISA Close(VISA resource name=w292, error in (no error)=w291) -> (error out=w294:errorcluster)
                n184 = call <vilib>:"Simple Error Handler.vi"("error in (no error)"=w294) -> ("error out"=→"error out 3":errorcluster)  [unwired: 4 in, 4 out]
                n185 = local read "VISA resource name 2"() -> (w311:string)
                n186 = call-poly "VISA Configure Serial Port"("VISA resource name"=w311, "timeout (10sec)"=u32 2000, "Enable Termination\nChar (T)"=FALSE ("Enable Termination\nChar (T)"), "baud rate (9600)"=u32 115200, "error in (no error)"="error in (no error) 4") -> ("VISA resource name out"=w315:refnum<visa-resource-name>, "error out"=w317:errorcluster)  [unwired: 9 in]
                n187 = property class="Instr"(reference=w315, error in=w317, "TermChar"=u8 10 ("Message Based Settings:Termination Character"), "ASRL End In"=w319, "ASRL End Out"=w320) -> (reference out=w316:refnum<visa-resource-name>, error out=w318:errorcluster)
                n188 = VISA Set I/O Buffer Size(VISA resource name=w316, error in (no error)=w318) -> (VISA resource name out=w322:refnum<visa-resource-name>, error out=w323:errorcluster)  [unwired: 2 in]
                n189 = VISA Flush I/O Buffer(VISA resource name=w322, error in (no error)=w323) -> (VISA resource name out=w325:refnum<visa-resource-name>, error out=w324:errorcluster)  [unwired: 1 in]
                n190 = case shown="No Error" w324 {
                  tunnel: w324 -> [w391 w431]
                  tunnel: w325 -> [w390 w432]
                  tunnel: [w389 w431] -> w288
                  tunnel: [w388 w432] -> w287
                  frame No Error {
                    w387 = 2 ("length (rest)")
                    # "Initialize Lens Driver"
                    n191 = local read "Calibration"() -> (w379:T2)
                    n192 = for {
                      tunnel: w390 -> [w429]
                      tunnel: [w426] -> w382
                      tunnel: string[] ["Start", "MwDA", "CrMA00", "CrMB00", "CrUA00", "CrUB00", "CrLA00", "CrLB00", "PwTA\u0002Ð\u0001@"] -> [w424] mode=indexing
                      tunnel: [w423] -> w381
                      shift-right: [w427] -> w383
                      shift-left: w379 -> [w428]
                      shift-right: [w425] -> w384
                      shift-left: w391 -> [w430]
                      n193 = call "write read Lens Driver.vi"("VISA resource name"=w429, "command"=w424, "Calibration"=w428, "error in (no error)"=w430) -> ("VISA resource name out"=w426:refnum<visa-resource-name>, "Calibration 2"=w427:T2, "Data"=w423:string, "error out"=w425:errorcluster)  [unwired: 4 in, 4 out]
                    }
                    n194 = String Subset(string=w381, offset (0)=w387, length (rest)=w387) -> (substring=w385:string)
                    n195 = Type Cast(type=u16 0 ("length (rest)"), x=w385) -> (*(type *) &x=w380:u16)
                    n196 = local write "ID"(w380) -> ()
                    n197 = while {
                      tunnel: [w393] -> w389
                      tunnel: [w394] -> w388
                      tunnel: w384 -> [w399]
                      tunnel: w383 -> [w398]
                      tunnel: w382 -> [w397]
                      stop <- w392 stop-if-true
                      # "When Send command is true, Current Ch A is sent to the Lens Driver, in the correct format. If answer exists it is displayed in Data. The update rate of the while loop is 2ms."
                      n198 = Wait Until Next ms Multiple(millisecond multiple=u32 2) -> ()  [unwired: 1 out]
                      n199 = case shown="True" TRUE ("Send command") {
                        tunnel: [w401 w422] -> w393
                        tunnel: w399 -> [w401 w421]
                        tunnel: w398 -> [_ w409]
                        tunnel: w397 -> [w400 w420]
                        tunnel: [w400 w410] -> w394
                        frame False {
                        }
                        frame True {
                          n200 = Unbundle By Name(w409) -> ("Max Current A"=w408:dbl)
                          n201 = Multiply(x=15.8, y="Potencia inicial lente izquierdo") -> (x*y=w406:dbl)
                          n202 = Add(x=-6.8, y=w406) -> (x+y=w404:dbl)
                          n203 = Divide(x=w404, y=w408) -> (x/y=w407:dbl)
                          n204 = Multiply(x=4096.0, y=w407) -> (x*y=w418:dbl)
                          n205 = To Word Integer(number=w418) -> (16bit integer=w417:i16)
                          n206 = Type Cast(x=w417) -> (*(type *) &x=w416:string)  [unwired: 1 in]
                          n207 = Concatenate Strings("Aw", w416) -> (w412:string)
                          n208 = local write "Command to Port"(w412) -> ()
                          n209 = call "write read Lens Driver.vi"("VISA resource name"=w420, "command"=w412, "Calibration"=w409, "error in (no error)"=w421) -> ("VISA resource name out"=w410:refnum<visa-resource-name>, "Calibration 2"=w414:T2, "OK"=w413:bool, "Data"=w411:string, "error out"=w422:errorcluster)  [unwired: 4 in, 3 out]
                          n210 = local write "VISA resource name out 2"(w410) -> ()
                          n211 = local write "Calibration 2"(w414) -> ()
                          n212 = local write "Data"(w411) -> ()
                          n213 = local write "OK"(w413) -> ()
                          "DPT INICIALES I" <- "Potencia inicial lente izquierdo"
                        }
                      }
                      n214 = local read "Parar adquisicion"() -> (w392:bool)
                    }
                  }
                  frame Error {
                  }
                }
                n215 = VISA Close(VISA resource name=w287, error in (no error)=w288) -> (error out=w290:errorcluster)
                n216 = call <vilib>:"Simple Error Handler.vi"("error in (no error)"=w290) -> ("error out"=→"error out 4":errorcluster)  [unwired: 4 in, 4 out]
              }
              frame 1 {
                # "Mensaje que pregunta si desea realizar el experimento\ncon un nuevo usuario o con el actual"
                # "Se vuelven 0 los valores del WL y de la potencia óptica y distancia"
                # "En esta opcion se activa el modo experimento"
                n217 = property on="Waveform length" class="WFChart (strict)"("History Data"=dbl[][] [[0.0]]) -> ()  [unwired: 2 in, 2 out]
                n218 = property on="Potencia Optica" class="WFChart (strict)"("History Data"=dbl[] [0.0]) -> ()  [unwired: 2 in, 2 out]
                n219 = Two Button Dialog(message="Con quien desea realizar los experimentos?", 1:"Nuevo voluntario" ("F button name (\"Cancel\")"), 2:"Voluntario actual" ("T button name (\"OK\")")) -> (T button?=w451:bool)
                n220 = flat-sequence {
                  tunnel: w451 -> [w464]
                  tunnel: [w463] -> w449
                  tunnel: w448 -> [w463]
                  tunnel: [w456] -> w436
                  tunnel: w435 -> [w456]
                  tunnel: [w474] -> w452
                  tunnel: [w476] -> w450
                  tunnel: w449 -> [w476]
                  tunnel: [w475] -> w446
                  tunnel: w445 -> [w475]
                  tunnel: [w473] -> w437
                  tunnel: w436 -> [w473]
                  tunnel: w452 -> [w488]
                  tunnel: w450 -> [w487]
                  tunnel: [w486] -> w447
                  tunnel: w446 -> [w485]
                  tunnel: [w484] -> w443
                  tunnel: [w483] -> w442
                  tunnel: [w482] -> w440
                  tunnel: [w481] -> w438
                  tunnel: w437 -> [w481]
                  tunnel: w443 -> [w534]
                  tunnel: w442 -> [w517]
                  tunnel: [w534] -> w441
                  tunnel: w440 -> [w520]
                  tunnel: [w513] -> w439
                  tunnel: w438 -> [w513]
                  tunnel: [w537] -> w444
                  tunnel: w441 -> [w537]
                  tunnel: w439 -> [w535]
                  frame #0 {
                    # "Se guardan los datos de un nuevo voluntario"
                    n221 = Not(x=w464) -> (.not. x?=w458:bool)
                    n222 = case shown="True" w458 {
                      tunnel: [w467 w472] -> w462
                      tunnel: [w466 w471] -> w461
                      tunnel: [w468 w470] -> w460
                      tunnel: [w465 w469] -> w459
                      frame False {
                        n223 = local read "Enfermedad visual"() -> (w467:string)
                        n224 = local read "Nombre"() -> (w468:string)
                        n225 = local read "Cedula"() -> (w465:string)
                        n226 = local read "Edad"() -> (w466:string)
                      }
                      frame True {
                        n227 = call "Registro voluntario"() -> ("Enfermedad visual"=w472:string, "Edad"=w471:string, "Cedula"=w469:string, "Nombre"=w470:string)  [unwired: 14 in, 2 out]
                      }
                    }
                    "Cedula" <- w459
                    "Nombre" <- w460
                    "Edad" <- w461
                    "Enfermedad visual" <- w462
                    n228 = local write "T button?"(FALSE ("T button?")) -> ()
                  }
                  frame #1 {
                    n229 = Two Button Dialog(message="Qué tipo de experimento desea realizar?", 1:"Nuevo Experimento" ("F button name (\"Cancel\")"), 2:"Experimento existente" ("T button name (\"OK\")")) -> (T button?=w477:bool)
                    n230 = Not(x=w477) -> (.not. x?=w474:bool)
                  }
                  frame #2 {
                    # "A partir de la seleccion del experimento, se obtiene la descripcion correspondiente que será guardada en el archivo"
                    n231 = case shown="False" w488 {
                      tunnel: w487 -> [w490 w508]
                      tunnel: [w490 w507] -> w486
                      tunnel: w485 -> [w492 w506]
                      tunnel: [w492 w505] -> w484
                      tunnel: [w493 w504] -> w483
                      tunnel: [w489 w503] -> w482
                      frame False {
                        n232 = call "Display Message to User"() -> ()  [unwired: 10 in, 2 out]
                        n233 = flat-sequence {
                          tunnel: [w494] -> w491
                          tunnel: w490 -> [w494]
                          tunnel: [w502] -> w493
                          tunnel: w492 -> [w501]
                          tunnel: ["Menu experimentos"] -> _
                          tunnel: w491 -> [w499]
                          tunnel: [w498] -> w489
                          frame #0 {
                            n234 = while {
                              stop <- w495 stop-if-true
                              # "El sistema se queda en el loop hasta que el usuario elija el experimento que desea realizar"
                              n235 = event shown="[0] \"Elegir menu Exp\": Value Change" {
                                selector: _ -> [_ _]
                                dyn-events: _ -> [_ _]
                                timeout: _ -> [_ _]
                                tunnel: [TRUE FALSE] -> w495
                                event "Elegir menu Exp": Value Change {
                                n236 = event-data() -> ()  [unwired: 1 in, 4 out]
                                }
                                event Timeout {
                                n237 = event-data() -> ()  [unwired: 1 in, 3 out]
                                }
                              }
                            }
                          }
                          frame #1 {
                            n238 = Index Array(array=w501, index="Menu experimentos") -> (element=w502:string)
                            n239 = Index Array(array=w499, index="Menu experimentos") -> (element=w498:string)
                          }
                        }
                        "Array" <- w490
                      }
                      frame True {
                        # "Se añade el nuevo experimento al menu de seleccion de experimentos"
                        # "Se guarda el nuevo experimento en el archivo que los contiene"
                        n240 = call "Nuevo experimento"() -> ("Descripcion"=w504:string, "Nombre"=w503:string)  [unwired: 16 in, 2 out]
                        n241 = Insert Into Array(array=w506, new element=w504) -> (w505:string[])  [unwired: 1 in]
                        n242 = Insert Into Array(array=w508, new element=w503) -> (w507:string[])  [unwired: 1 in]
                        n243 = property on="Menu experimentos" class="Ring (strict)"("Strings []"=w507) -> ()  [unwired: 2 in, 2 out]
                        n244 = Insert Into Array(array=string[] [], new element #1=w503, new element #2=w504) -> (w510:string[])  [unwired: 1 in]
                        n245 = call-poly <vilib>:"Write Delimited Spreadsheet.vi"("file path (dialog if empty)"=path "C:/Users/TGM1603/Documents/LabVIEW Data/Experimentos_realizados", "1D data"=w510, "append to file? (new file:F)"=TRUE) -> ()  [unwired: 11 in, 2 out]
                      }
                    }
                  }
                  frame #3 {
                    # "Se guardan los datos generales del experimento en el archivo de excel"
                    n246 = local read "factor decimacion"() -> (w516:i32)
                    n247 = local read "Enfermedad visual"() -> (w519:string)
                    n248 = local read "Cedula"() -> (w521:string)
                    n249 = local read "Edad"() -> (w518:string)
                    n250 = local read "Nombre"() -> (w522:string)
                    n251 = Get Date/Time In Seconds() -> (seconds since 1Jan1904=w533:timestamp)
                    n252 = Path To String(path="Carpeta") -> (string=w529:string)
                    n253 = Format Date/Time String(time format string (%c)="_%d-%m-%y_%H-%M", seconds (now)=w533) -> (date/time string=w531:string)  [unwired: 1 in]
                    n254 = Number To Fractional String(number=w516, precision (6)=i16 0) -> (F-format string=w515:string)  [unwired: 2 in]
                    n255 = local read "Cedula"() -> (w525:string)
                    n256 = Concatenate Strings(w529, "\\" ("string"), w525, w531, "_" ("string"), w520, ".xlsx" ("string")) -> (w527:string)
                    n257 = String To Path(string=w527) -> (path=w526:path)
                    "path" <- w526
                    n258 = call "MS Office Report"("Path to Save Report"=w526, "Cedula"=w521, "decimacion"=w515, "Edad"=w518, "Enfermedad"=w519, "Exp_nombre"=w520, "Experimento"=w517, "Nombre"=w522) -> ()  [unwired: 18 in, 2 out]
                    "Nombre 2" <- w520
                  }
                  frame #4 {
                    n259 = while {
                      shift-right: [w539] -> _
                      shift-left: enum16{"Inicio", "Tomar datos", ""}."Inicio" -> [w541]
                      tunnel: w535 -> [w538]
                      stop <- w540 stop-if-true
                      n260 = case shown="\"Tomar datos\"" w541 {
                        tunnel: [w542 w553] -> w539
                        tunnel: w538 -> [_ w548]
                        frame "Inicio", Default {
                          # "Se chequea si el usuario ha presionado el boton de comenzar el experimento. Si no lo ha hecho, se queda en este estado (0).\n Cuando lo presiona, pasa al estado de adquirir datios (1) ."
                          n261 = Select(t=enum16{"Inicio", "Tomar datos", ""}."Tomar datos", s="Iniciar experimento", f=enum16{"Inicio", "Tomar datos", ""}."Inicio") -> (s? t:f=w542:enum16{"Inicio", "Tomar datos", ""})
                        }
                        frame "Tomar datos" {
                          n262 = flat-sequence {
                            tunnel: [w631] -> w552
                            tunnel: [w630] -> w551
                            tunnel: [w629] -> w550
                            tunnel: [w628] -> w549
                            tunnel: w548 -> [w623]
                            tunnel: [w606] -> w547
                            tunnel: [w588] -> w546
                            tunnel: w552 -> [w886]
                            tunnel: w551 -> [w885]
                            tunnel: w550 -> [w884]
                            tunnel: w549 -> [w883]
                            tunnel: w547 -> [w880]
                            tunnel: w546 -> [w881]
                            tunnel: [enum16{"Inicio", "Tomar datos", ""}."Inicio"] -> w553
                            frame #0 {
                              w575 = u16 0 items=["None", "Last Bit", "TermChar", "Break"] ("Serial Settings:End Mode for Writes")
                              w576 = u16 2 items=["None", "Last Bit", "TermChar"] ("Serial Settings:End Mode for Reads")
                              w597 = u16 0 items=["None", "Last Bit", "TermChar", "Break"] ("Serial Settings:End Mode for Writes")
                              w598 = u16 2 items=["None", "Last Bit", "TermChar"] ("Serial Settings:End Mode for Reads")
                              w621 = 100  # max queue size
                              # "[9] Se unen en una sola matriz los vectores de tiempo, distancia, potencia derecha y potencia izquierda."
                              # "[9]"
                              # "[12] Se unen en una sola matriz, los vectores de  tiempo de la señal EMG, amplitud de la señal EMG, tiempo de potencia óptica, distancia, potencia óptica derecha y potencia óptica izquierda, en ese orden."
                              # "[8]"
                              # "[7]"
                              # "[6]"
                              # "[5]"
                              # "Se usan registros de desplazamiento para concatenar en un solo vector los datos que se obtienen en cada iteracion. Así en \n[1] Se guarda la potencia del lente derecho.\n[2] Por medio de variables locales, se guarda la distancia que se obtuvo en el bloque de distancia.\n[3]  Por medio de variables locales, se guarda la potencia del lente izquierdo que se obtuvo en el bloque de control de potencia del lente izquierdo.\n[4] Se guarda el tiempo actual.\n[5] Se pasa el vector de de potencia derecha a variable a string con 2 cifras significativas. \n[6] Se ajusta el vector del tiempo para que se muestre un tiempo relativo, es decir, en donde el primer dato sea 0 y en los demas se aumente un dt.  Además, se pasa el vector a variable a string con 5 cifras significativas.\n[7] Se pasa el vector de de distancia a variable a string con 0 cifras significativas. \n[8] Se pasa el vector de de potencia izquierda a variable a string con 2 cifras significativas."
                              # "En esta cola se guarda los datos de la señal EMG\nEn el bloque de adquisición los añade al adquirirlos y  en el de procesamiento los elimina al procesarlos ."
                              # "Initialize VISA port with correct parameters"
                              # "Initialize VISA port with correct parameters"
                              # "Close VISA port after program stop. Otherwise this port is blocked."
                              # "Se adquiere la señal del circuito de adquisicion, en donde se define la frecuencia de muestreo y el factor de decimacion.\n[1] Se inicializa el canal de adquisicion\n[2] Se ajusta el canal para que lea muestras continuas y apartir de estas prooduzca waveform data.\n[3]  Se obtiene los datos de la señal: la amplitud Y, el tiempo de inicio y el delta t.\n[4] Se decima el vector de amplitud. \n[5] Se usan registros de desplazamiento para concatenenar en un solo vector los datos de la amplitud que se obtienen en cada iteración. \n[6] Se obtiene el vector del tiempo."
                              # "[11] Los vectores de amplitud y tiempo se transforman a formato texto con 4 y 5 cifras significativas respectivamente y se unen para formar un vector de 2 columnas."
                              # "[9] Se ajusta el vector del tiempo para que se muestre un tiempo relativo, es decir, en donde el primer dato sea 0 y en los demas se aumente un dt. \n[10] Se extrae el primer elemento del vector ya que este siempre es 0 y no aporta información"
                              # "[12]"
                              # "[11]"
                              # "[10]"
                              # "[9]"
                              # "[8] Se guarda la fecha/hora en que se inicio el experimento"
                              # "[7] Se usan registros de desplazamiento para concatenar en un solo vector los datos del tiempo que se obtienen en cada iteracion."
                              # "[1]"
                              n263 = local read "error in (no error)"() -> (w593:errorcluster)
                              n264 = local read "VISA resource name"() -> (w592:string)
                              n265 = local read "VISA resource name 2"() -> (w571:string)
                              n266 = call-poly "VISA Configure Serial Port"("VISA resource name"=w592, "timeout (10sec)"=u32 2000, "Enable Termination\nChar (T)"=FALSE ("Enable Termination\nChar (T)"), "baud rate (9600)"=u32 115200, "error in (no error)"=w593) -> ("VISA resource name out"=w602:refnum<visa-resource-name>, "error out"=w600:errorcluster)  [unwired: 9 in]
                              n267 = call-poly "VISA Configure Serial Port"("VISA resource name"=w571, "timeout (10sec)"=u32 2000, "Enable Termination\nChar (T)"=FALSE ("Enable Termination\nChar (T)"), "baud rate (9600)"=u32 115200, "error in (no error)"="error in (no error) 5") -> ("VISA resource name out"=w580:refnum<visa-resource-name>, "error out"=w578:errorcluster)  [unwired: 9 in]
                              n268 = property class="Instr"(reference=w602, error in=w600, "TermChar"=u8 10 ("Message Based Settings:Termination Character"), "ASRL End In"=w598, "ASRL End Out"=w597) -> (reference out=w601:refnum<visa-resource-name>, error out=w599:errorcluster)
                              n269 = property class="Instr"(reference=w580, error in=w578, "TermChar"=u8 10 ("Message Based Settings:Termination Character"), "ASRL End In"=w576, "ASRL End Out"=w575) -> (reference out=w579:refnum<visa-resource-name>, error out=w577:errorcluster)
                              n270 = VISA Set I/O Buffer Size(VISA resource name=w601, error in (no error)=w599) -> (VISA resource name out=w595:refnum<visa-resource-name>, error out=w594:errorcluster)  [unwired: 2 in]
                              n271 = invoke on="Parar adquisicion" class="Bool (strict)" method="Reinit To Default"() -> ()  [unwired: 3 in, 3 out]
                              n272 = VISA Set I/O Buffer Size(VISA resource name=w579, error in (no error)=w577) -> (VISA resource name out=w573:refnum<visa-resource-name>, error out=w572:errorcluster)  [unwired: 2 in]
                              n273 = VISA Flush I/O Buffer(VISA resource name=w595, error in (no error)=w594) -> (VISA resource name out=w591:refnum<visa-resource-name>, error out=w590:errorcluster)  [unwired: 1 in]
                              n274 = VISA Flush I/O Buffer(VISA resource name=w573, error in (no error)=w572) -> (VISA resource name out=w569:refnum<visa-resource-name>, error out=w568:errorcluster)  [unwired: 1 in]
                              n275 = Obtain Queue(max queue size (-1, unlimited)=w621, element data type="Cola tipo 2") -> (queue out=w620:refnum<queue>)  [unwired: 3 in, 2 out]
                              n276 = Enqueue Element(queue=w623, element=0.0) -> (queue out=w625:refnum<queue>)  [unwired: 2 in, 2 out]
                              n277 = case shown="No Error" w568 {
                                tunnel: w568 -> [w663 w720]
                                tunnel: w569 -> [w662 w721]
                                tunnel: [w661 w720] -> w558
                                tunnel: [w660 w721] -> w557
                                tunnel: [w650 dbl[] [-30.0]] -> _
                                frame No Error {
                                w659 = 2 ("length (rest)")
                                # "Bloque de control del izquierdo. Se explica en el caso 0 de visualziación general"
                                # "Initialize Lens Driver"
                                n278 = local read "Calibration"() -> (w651:T2)
                                n279 = for {
                                tunnel: w662 -> [w717]
                                tunnel: [w714] -> w654
                                tunnel: string[] ["Start", "MwDA", "CrMA00", "CrMB00", "CrUA00", "CrUB00", "CrLA00", "CrLB00", "PwTA\u0002Ð\u0001@"] -> [w712] mode=indexing
                                tunnel: [w711] -> w653
                                shift-right: [w715] -> w655
                                shift-left: w651 -> [w716]
                                shift-right: [w713] -> w656
                                shift-left: w663 -> [w718]
                                n280 = call "write read Lens Driver.vi"("VISA resource name"=w717, "command"=w712, "Calibration"=w716, "error in (no error)"=w718) -> ("VISA resource name out"=w714:refnum<visa-resource-name>, "Calibration 2"=w715:T2, "Data"=w711:string, "error out"=w713:errorcluster)  [unwired: 4 in, 4 out]
                                }
                                n281 = String Subset(string=w653, offset (0)=w659, length (rest)=w659) -> (substring=w657:string)
                                n282 = Type Cast(type=u16 0 ("length (rest)"), x=w657) -> (*(type *) &x=w652:u16)
                                n283 = local write "ID"(w652) -> ()
                                n284 = while {
                                tunnel: [w668] -> w661
                                tunnel: [w669] -> w660
                                tunnel: w656 -> [w674]
                                tunnel: w655 -> [w673]
                                tunnel: w654 -> [w672]
                                shift-right: [w665] -> w650
                                shift-left: _ -> [w666]
                                stop <- w667 stop-if-true
                                # "When Send command is true, Current Ch A is sent to the Lens Driver, in the correct format. If answer exists it is displayed in Data. The update rate of the while loop is 2ms."
                                n285 = case shown="True" TRUE ("Send command") {
                                tunnel: [w680 w703] -> w668
                                tunnel: w674 -> [w680 w702]
                                tunnel: w673 -> [_ w683]
                                tunnel: w672 -> [w679 w701]
                                tunnel: [w679 w694] -> w669
                                tunnel: [dbl[] [-20.0] w693] -> w665
                                tunnel: w666 -> [_ w692]
                                frame False {
                                }
                                frame True {
                                n286 = local read "Potencia inicial lente izquierdo"() -> (w691:dbl)
                                n287 = local read "DPT dif."() -> (w690:dbl)
                                n288 = Add(x=w690, y=w691) -> (x+y=w686:dbl)
                                n289 = Absolute Value(x=w686) -> (abs(x)=w688:dbl)
                                n290 = Greater Or Equal?(x=6.0, y=w688) -> (x >= y?=w687:bool)
                                n291 = case shown="False" w687 {
                                tunnel: w686 -> [w706 w710]
                                tunnel: [w704 w710] -> w684
                                frame False {
                                n292 = Greater Or Equal?(x=u16 0, y=w706) -> (x >= y?=w707:bool)
                                n293 = case shown="False" w707 {
                                tunnel: [i16 6 ("x") i16 -6 ("x")] -> w704
                                frame False {
                                }
                                frame True {
                                }
                                }
                                }
                                frame True {
                                }
                                }
                                "Potencia izquierdo" <- w684
                                n294 = Unbundle By Name(w683) -> ("Max Current A"=w682:dbl)
                                n295 = call "potencia a corriente.vi"("Max current A"=w682, "Potencia"=w684) -> ("Corriente"=w685:dbl)
                                n296 = To Word Integer(number=w685) -> (16bit integer=w700:i16)
                                n297 = Type Cast(x=w700) -> (*(type *) &x=w699:string)  [unwired: 1 in]
                                n298 = Concatenate Strings("Aw", w699) -> (w696:string)
                                n299 = local write "Command to Port"(w696) -> ()
                                n300 = call "write read Lens Driver.vi"("VISA resource name"=w701, "command"=w696, "Calibration"=w683, "error in (no error)"=w702) -> ("VISA resource name out"=w694:refnum<visa-resource-name>, "Calibration 2"=w698:T2, "OK"=w697:bool, "Data"=w695:string, "error out"=w703:errorcluster)  [unwired: 4 in, 3 out]
                                n301 = local write "VISA resource name 2"(w694) -> ()
                                n302 = local write "Calibration 2"(w698) -> ()
                                n303 = local write "Data"(w695) -> ()
                                n304 = local write "OK"(w697) -> ()
                                n305 = Build Array (concatenate)(w692, w684) -> (w693:dbl[])
                                }
                                }
                                n306 = Wait Until Next ms Multiple(millisecond multiple=u32 10) -> ()  [unwired: 1 out]
                                n307 = local read "Parar adquisicion"() -> (w667:bool)
                                n308 = event shown="[0] \"Restablecer Iniciales\": Value Change" {
                                selector: _ -> [_ _]
                                dyn-events: _ -> [_ _]
                                timeout: 100 -> [_ _]
                                event "Restablecer Iniciales": Value Change {
                                n309 = event-data() -> ()  [unwired: 1 in, 3 out]
                                n310 = local read "Potencia inicial lente izquierdo"() -> (w675:dbl)
                                n311 = local read "Potencia inicial lente derecho"() -> (w676:dbl)
                                n312 = local write "Potencia izquierdo"(w675) -> ()
                                n313 = local write "Potencia derecho"(w676) -> ()
                                n314 = local write "DPT dif."(0.0 ("DPT dif.")) -> ()
                                }
                                event Timeout {
                                n315 = event-data() -> ()  [unwired: 1 in, 3 out]
                                }
                                }
                                }
                                }
                                frame Error {
                                }
                              }
                              n316 = case shown="No Error" w590 {
                                tunnel: w590 -> [w741 w831]
                                tunnel: w591 -> [w740 w832]
                                tunnel: [w739 w831] -> w618
                                tunnel: [w738 w832] -> w617
                                tunnel: [w727 dbl[] [-1.0]] -> w610
                                tunnel: [w726 dbl[] [-30.0]] -> w562
                                tunnel: [w724 dbl[] [-30.0]] -> w565
                                frame No Error {
                                w737 = 2 ("length (rest)")
                                # "Bloque de control del lente derecho. Se explica en el caso 0 de visualziación general"
                                # "Initialize Lens Driver"
                                n317 = local read "Calibration"() -> (w729:T2)
                                n318 = for {
                                tunnel: w740 -> [w826]
                                tunnel: [w823] -> w732
                                tunnel: string[] ["Start", "MwDA", "CrMA00", "CrMB00", "CrUA00", "CrUB00", "CrLA00", "CrLB00", "PwTA\u0002Ð\u0001@"] -> [w821] mode=indexing
                                tunnel: [w820] -> w731
                                shift-right: [w824] -> w733
                                shift-left: w729 -> [w825]
                                shift-right: [w822] -> w734
                                shift-left: w741 -> [w827]
                                n319 = call "write read Lens Driver.vi"("VISA resource name"=w826, "command"=w821, "Calibration"=w825, "error in (no error)"=w827) -> ("VISA resource name out"=w823:refnum<visa-resource-name>, "Calibration 2"=w824:T2, "Data"=w820:string, "error out"=w822:errorcluster)  [unwired: 4 in, 4 out]
                                }
                                n320 = String Subset(string=w731, offset (0)=w737, length (rest)=w737) -> (substring=w735:string)
                                n321 = Type Cast(type=u16 0 ("length (rest)"), x=w735) -> (*(type *) &x=w730:u16)
                                n322 = local write "ID"(w730) -> ()
                                n323 = while {
                                tunnel: [w754] -> w739
                                tunnel: [w755] -> w738
                                tunnel: w734 -> [w760]
                                tunnel: w733 -> [w759]
                                tunnel: w732 -> [w758]
                                shift-right: [w747] -> w727
                                shift-left: dbl[] [0.0] -> [w748]
                                shift-right: [w742] -> w726
                                shift-left: dbl[] [0.0] -> [w752]
                                shift-right: [w745] -> w724
                                shift-left: dbl[] [0.0] -> [w744]
                                stop <- w753 stop-if-true
                                # "[4]"
                                # "[3]"
                                # "When Send command is true, Current Ch A is sent to the Lens Driver, in the correct format. If answer exists it is displayed in Data. The update rate of the while loop is 2ms."
                                n324 = Wait Until Next ms Multiple(millisecond multiple=u32 10) -> ()  [unwired: 1 out]
                                n325 = case shown="True" TRUE ("Send command") {
                                tunnel: [w767 w786] -> w754
                                tunnel: w760 -> [w767 w785]
                                tunnel: w759 -> [_ w770]
                                tunnel: w758 -> [w766 w784]
                                tunnel: [w766 w776] -> w755
                                tunnel: [dbl[] [-20.0] w775] -> w742
                                tunnel: w752 -> [_ w774]
                                frame False {
                                }
                                frame True {
                                # "[1]"
                                n326 = local read "number"() -> (w781:u32)
                                n327 = local read "Potencia inicial lente derecho"() -> (w773:dbl)
                                n328 = case shown="2" w781 {
                                tunnel: [w787 w796 w811] -> w772
                                tunnel: w773 -> [w789 w791 w806]
                                tunnel: w773 -> [_ w790 w805]
                                frame 0, Default {
                                n329 = local read "DPT dif."() -> (w788:dbl)
                                n330 = Add(x=w789, y=w788) -> (x+y=w787:dbl)
                                }
                                frame 1 {
                                n331 = local read "DPT dif."() -> (w792:dbl)
                                n332 = Add(x=w791, y=w792) -> (x+y=w793:dbl)
                                n333 = Less Or Equal?(x=w793, y=6.0) -> (x <= y?=w795:bool)
                                n334 = case shown="True" w795 {
                                tunnel: [w798 w802] -> w796
                                tunnel: w790 -> [w797 w801]
                                frame False {
                                n335 = local read "DPT dif."() -> (w799:dbl)
                                n336 = Add(x=w797, y=w799) -> (x+y=w798:dbl)
                                }
                                frame True {
                                n337 = local read "DPT dif."() -> (w803:dbl)
                                n338 = local read "Incremento"() -> (w800:dbl)
                                n339 = Add(x=w803, y=w800) -> (x+y=w804:dbl)
                                n340 = local write "DPT dif."(w804) -> ()
                                n341 = Add(x=w801, y=w804) -> (x+y=w802:dbl)
                                }
                                }
                                }
                                frame 2 {
                                n342 = local read "DPT dif."() -> (w810:dbl)
                                n343 = Add(x=w810, y=w806) -> (x+y=w807:dbl)
                                n344 = Greater Or Equal?(x=w807, y=-6.0) -> (x >= y?=w808:bool)
                                n345 = case shown="True" w808 {
                                tunnel: [w813 w817] -> w811
                                tunnel: w805 -> [w812 w816]
                                frame False {
                                n346 = local read "DPT dif."() -> (w814:dbl)
                                n347 = Add(x=w812, y=w814) -> (x+y=w813:dbl)
                                }
                                frame True {
                                n348 = local read "DPT dif."() -> (w819:dbl)
                                n349 = local read "Incremento"() -> (w815:dbl)
                                n350 = Subtract(x=w819, y=w815) -> (x-y=w818:dbl)
                                n351 = local write "DPT dif."(w818) -> ()
                                n352 = Add(x=w816, y=w818) -> (x+y=w817:dbl)
                                }
                                }
                                }
                                }
                                "Potencia derecho" <- w772
                                n353 = Unbundle By Name(w770) -> ("Max Current A"=w769:dbl)
                                n354 = call "potencia a corriente.vi"("Max current A"=w769, "Potencia"=w772) -> ("Corriente"=w771:dbl)
                                n355 = To Word Integer(number=w771) -> (16bit integer=w783:i16)
                                n356 = Type Cast(x=w783) -> (*(type *) &x=w782:string)  [unwired: 1 in]
                                n357 = Concatenate Strings("Aw", w782) -> (w778:string)
                                n358 = local write "Command to Port"(w778) -> ()
                                n359 = call "write read Lens Driver.vi"("VISA resource name"=w784, "command"=w778, "Calibration"=w770, "error in (no error)"=w785) -> ("VISA resource name out"=w776:refnum<visa-resource-name>, "Calibration 2"=w780:T2, "OK"=w779:bool, "Data"=w777:string, "error out"=w786:errorcluster)  [unwired: 4 in, 3 out]
                                n360 = local write "VISA resource name out"(w776) -> ()
                                n361 = local write "Calibration 2"(w780) -> ()
                                n362 = local write "Data"(w777) -> ()
                                n363 = local write "OK"(w779) -> ()
                                n364 = Build Array (concatenate)(w774, w772) -> (w775:dbl[])
                                }
                                }
                                "Potencia Optica" <- w742
                                n365 = local read "Parar adquisicion"() -> (w753:bool)
                                n366 = local read "Potencia izquierdo"() -> (w743:dbl)
                                n367 = property on="Potencia optica" class="WFChart (strict)"("YScale.ScaleFit"="Auto scale Y") -> ()  [unwired: 2 in, 2 out]
                                n368 = Get Date/Time In Seconds() -> (seconds since 1Jan1904=w749:timestamp)
                                n369 = To Double Precision Float(number=w749) -> (double precision float=w746:dbl)
                                n370 = property on="Potencia Optica" class="WFChart (strict)"("XScale.ScaleFit"="Auto scale X") -> ()  [unwired: 2 in, 2 out]
                                n371 = Build Array (concatenate)(w748, w746) -> (w747:dbl[])
                                n372 = case shown="0, Default" "Auto scale Y" {
                                frame 0, Default {
                                n373 = property on="Potencia Optica" class="WFChart (strict)"("YScale.Maximum"="Escala Y max") -> ()  [unwired: 2 in, 2 out]
                                n374 = property on="Potencia Optica" class="WFChart (strict)"("YScale.Minimum"="Escala Y min") -> ()  [unwired: 2 in, 2 out]
                                }
                                frame 1 {
                                }
                                }
                                n375 = Build Array (concatenate)(w744, w743) -> (w745:dbl[])
                                n376 = case shown="0, Default" "Auto scale X" {
                                frame 0, Default {
                                n377 = property on="Potencia Optica" class="WFChart (strict)"("XScale.Maximum"="Escala X max") -> ()  [unwired: 2 in, 2 out]
                                n378 = property on="Potencia Optica" class="WFChart (strict)"("XScale.Minimum"="Escala X min") -> ()  [unwired: 2 in, 2 out]
                                }
                                frame 1 {
                                }
                                }
                                }
                                }
                                frame Error {
                                }
                              }
                              n379 = while {
                                tunnel: w625 -> [w843]
                                shift-right: [w845] -> _
                                shift-left: dbl[] [0.0] -> [w851]
                                shift-right: [w844] -> _
                                shift-left: u32[] [0] -> [w846]
                                tunnel: [w843] -> _
                                tunnel: w620 -> [w835]
                                stop <- w834 stop-if-true
                                # "Bloque de procesamiento.  Se explica en el caso 0 de visualización general"
                                n380 = local read "WL"() -> (w842:dbl)
                                n381 = local read "Parar adquisicion"() -> (w834:bool)
                                n382 = local read "Limite superior WL"() -> (w839:dbl)
                                n383 = call "waveform_length.vi"("WL"=w842, "Cola WL"=w843, "Datos entrada"=w835) -> ("WL 2"=w850:dbl)
                                n384 = local read "Limite inferior WL"() -> (w841:dbl)
                                n385 = local write "WL"(w850) -> ()
                                n386 = Build Array (concatenate)(w851, w850) -> (w845:dbl[])
                                n387 = In Range and Coerce(upper limit=w839, x=w850, lower limit=w841) -> (In Range?=w848:bool)  [unwired: 1 out]
                                n388 = Greater?(x=w850, y=w839) -> (0:w849:bool)
                                n389 = local read "Escala autom. X"() -> (w836:u8)
                                n390 = local read "Escala autom. Y"() -> (w837:u8)
                                n391 = Build Array(w849, w848) -> (w847:bool[])
                                n392 = Boolean Array To Number(Boolean array=w847) -> (number=w840:u32)
                                n393 = local write "number"(w840) -> ()
                                n394 = Build Array (concatenate)(w846, w840) -> (w844:u32[])
                                n395 = Build Array(w845, w844) -> (w838:dbl[][])
                                n396 = Transpose 2D Array(2D array=w838) -> (transposed array=w833:dbl[][])
                                n397 = local write "Waveform length"(w833) -> ()
                                n398 = property on="Waveform length" class="WFChart (strict)"("XScale.ScaleFit"=w836) -> ()  [unwired: 2 in, 2 out]
                                n399 = property on="Waveform length" class="WFChart (strict)"("YScale.ScaleFit"=w837) -> ()  [unwired: 2 in, 2 out]
                                n400 = case shown="0, Default" w837 {
                                frame 0, Default {
                                n401 = local read "Maximo escala Y"() -> (w855:dbl)
                                n402 = local read "Minimo escala Y"() -> (w854:dbl)
                                n403 = property on="Waveform length" class="WFChart (strict)"("YScale.Maximum"=w855) -> ()  [unwired: 2 in, 2 out]
                                n404 = property on="Waveform length" class="WFChart (strict)"("YScale.Minimum"=w854) -> ()  [unwired: 2 in, 2 out]
                                }
                                frame 1 {
                                }
                                }
                                n405 = case shown="0, Default" w836 {
                                frame 0, Default {
                                n406 = local read "Minimo escala X"() -> (w853:dbl)
                                n407 = local read "Maximo escala X"() -> (w852:dbl)
                                n408 = property on="Waveform length" class="WFChart (strict)"("XScale.Minimum"=w853) -> ()  [unwired: 2 in, 2 out]
                                n409 = property on="Waveform length" class="WFChart (strict)"("XScale.Maximum"=w852) -> ()  [unwired: 2 in, 2 out]
                                }
                                frame 1 {
                                }
                                }
                              }
                              n410 = while {
                                tunnel: [w874] -> w648
                                shift-right: [w873] -> w630
                                shift-left: _ -> [w872]
                                shift-right: [w864] -> w633
                                shift-left: dbl[] [0.0] -> [w869]
                                shift-right: [w865] -> w638
                                shift-left: dbl[] [0.0] -> [w866]
                                tunnel: w620 -> [w859]
                                i -> [w875]
                                stop <- w856 stop-if-true
                                # "[7]"
                                # "[6]"
                                # "[5]"
                                # "[4]"
                                # "[3]"
                                # "[2]"
                                n411 = local read "Parar adquisicion"() -> (w856:bool)
                                n412 = call-poly <vilib>:"Index Waveform Array.vi"("index"=0, "waveform array"=waveform(dbl)[] []) -> ("waveform"=w868:waveform(dbl))  [unwired: 8 in, 1 out]
                                n413 = Unbundle By Name(w868) -> ("Y"=w860:dbl[], "t0"=w874:timestamp)  [unwired: 1 out]
                                n414 = call-poly <vilib>:"Decimate (continuous).vi"("averaging"=TRUE, "decimating factor"="factor decimacion", "X"=w860) -> ("Decimated Array"=w858:dbl[])  [unwired: 7 in, 1 out]
                                n415 = Lossy Enqueue Element(queue=w859, element=w858) -> ()  [unwired: 1 in, 4 out]
                                n416 = Build Array (concatenate)(w869, w858) -> (w864:dbl[])
                                n417 = case shown="1" w875 {
                                tunnel: w874 -> [_ w879]
                                tunnel: [w877 w878] -> w873
                                tunnel: w872 -> [w877 _]
                                frame 0, Default {
                                }
                                frame 1 {
                                # "[8]"
                                n418 = Format Date/Time String(seconds (now)=w879) -> (date/time string=w878:string)  [unwired: 2 in]
                                }
                                }
                                n419 = local read "factor decimacion"() -> (w861:i32)
                                n420 = call-poly <vilib>:"Get Waveform Time Array.vi"("waveform in"=w868) -> ("X array"=w867:timestamp[])  [unwired: 9 in, 1 out]
                                n421 = To Double Precision Float(number=w867) -> (double precision float=w863:dbl[])
                                n422 = call-poly <vilib>:"Decimate (single shot).vi"("decimating factor"=w861, "X"=w863) -> ("Decimated Array"=w862:dbl[])  [unwired: 8 in, 1 out]
                                n423 = Build Array (concatenate)(w866, w862) -> (w865:dbl[])
                              }
                              n424 = Index Array(array=w638, index=1) -> (element=w637:dbl)
                              n425 = Subtract(x=w638, y=w637) -> (x-y=w635:dbl[])
                              n426 = Delete From Array(array=w633, index=0) -> (array with subset deleted=w643:dbl[])  [unwired: 1 in, 1 out]
                              n427 = Delete From Array(array=w635, index=0) -> (array with subset deleted=w642:dbl[])  [unwired: 1 in, 1 out]
                              n428 = local read "path"() -> (w631:path)
                              n429 = Format Date/Time String(seconds (now)=w648) -> (date/time string=w629:string)  [unwired: 2 in]
                              n430 = Number To Fractional String(use system decimal point (T)=FALSE, number=w643, precision (6)=i16 4) -> (F-format string=w586:string[])  [unwired: 1 in]
                              n431 = Number To Fractional String(use system decimal point (T)=FALSE, number=w642, precision (6)=i16 5) -> (F-format string=w587:string[])  [unwired: 1 in]
                              n432 = Build Array(w587, w586) -> (w641:string[][])
                              n433 = Transpose 2D Array(2D array=w641) -> (transposed array=w628:string[][])
                              n434 = Delete From Array(array=w562, index=0) -> (array with subset deleted=w561:dbl[])  [unwired: 1 in, 1 out]
                              n435 = Index Array(array=w610, index=1) -> (element=w615:dbl)
                              n436 = Delete From Array(array=w565, index=0) -> (array with subset deleted=w564:dbl[])  [unwired: 1 in, 1 out]
                              n437 = VISA Close(VISA resource name=w557, error in (no error)=w558) -> (error out=w556:errorcluster)
                              n438 = Subtract(x=w610, y=w615) -> (x-y=w609:dbl[])
                              n439 = Number To Fractional String(use system decimal point (T)=FALSE, number=w561, precision (6)=i16 2) -> (F-format string=w584:string[])  [unwired: 1 in]
                              n440 = VISA Close(VISA resource name=w617, error in (no error)=w618) -> (error out=w619:errorcluster)
                              n441 = call <vilib>:"Simple Error Handler.vi"("error in (no error)"=w556) -> ("error out"=w555:errorcluster)  [unwired: 4 in, 4 out]
                              n442 = Delete From Array(array=w609, index=0) -> (array with subset deleted=w614:dbl[])  [unwired: 1 in, 1 out]
                              n443 = call <vilib>:"Simple Error Handler.vi"("error in (no error)"=w619) -> ("error out"=w616:errorcluster)  [unwired: 4 in, 4 out]
                              n444 = Number To Fractional String(use system decimal point (T)=FALSE, number=w564, precision (6)=i16 2) -> (F-format string=w554:string[])  [unwired: 1 in]
                              n445 = local write "error out"(w616) -> ()
                              n446 = local write "error out"(w555) -> ()
                              n447 = Number To Fractional String(use system decimal point (T)=FALSE, number=w614, precision (6)=i16 5) -> (F-format string=w585:string[])  [unwired: 1 in]
                              n448 = Build Array(w587, w586, w585, w554, w584) -> (w559:string[][])
                              n449 = Transpose 2D Array(2D array=w559) -> (transposed array=w588:string[][])
                              n450 = Build Array(w585, w554, w584) -> (w606:string[][])
                            }
                            frame #1 {
                              # "[13]"
                              # "[13] En esta case structure, se decide que datos se van a guardar. Esto lo hace el SUBVI llamado guardar datos de amplitud y tiempo."
                              n451 = Transpose 2D Array(2D array=w880) -> (transposed array=w882:string[][])
                              n452 = call <vilib>:"Three Button Dialog.vi"("Right Button Text (\"Cancel\")"="Señal EMG, potencia optica y distancia" ("Right Button Text (\"Cancel\")"), "Center Button Text (\"No\")"="Potencia optica" ("Center Button Text (\"No\")"), "Left Button Text (\"Yes\")"="Señal EMG" ("Left Button Text (\"Yes\")"), "message"="Elija que datos desea guardar") -> ("Which Button?"=w887:T3)  [unwired: 7 in]
                              n453 = case shown="\"Center Button\"" w887 {
                                tunnel: w886 -> [w896 w901 w904]
                                tunnel: w885 -> [w895 w900 w905]
                                tunnel: w884 -> [w894 w899 w906]
                                tunnel: w883 -> [w893 _ _]
                                tunnel: w882 -> [_ w898 _]
                                tunnel: w881 -> [_ _ w902]
                                frame "Left Button", Default {
                                # "Se guarda solo la señal EMG y su tiempo de adquisición."
                                n454 = call "Guardar datos de Amplitud y Tiempo.vi"("path"=w896, "Hora inicio"=w895, "Hora fin"=w894, "Datos experimento"=w893, "column headers"=string[] ["Tiempo(s)", "Amplitud(V)"]) -> ()  [unwired: 1 in]
                                }
                                frame "Center Button" {
                                # "Se guarda la potenica del lente derecho, del lente izquierdo, la distancia y el tiempo de estas variables."
                                n455 = call "Guardar datos de Amplitud y Tiempo.vi"("path"=w901, "Hora inicio"=w900, "Hora fin"=w899, "Datos experimento"=w898, "column headers"=string[] ["Tiempo(s)", "Distancia (cm)", "Potencia Optica derecho", "Potencia optica izquierdo"]) -> ()  [unwired: 1 in]
                                }
                                frame "Right Button" {
                                # "Se guarda el tiempo de adquisición así como la amplitud de la señal EMG,  la potenica del lente derecho, del lente izquierdo, la distancia y el tiempo de estas variables."
                                n456 = call "Guardar datos de Amplitud y Tiempo.vi"("path"=w904, "Hora inicio"=w905, "Hora fin"=w906, "Datos experimento"=w902, "column headers"=string[] ["Tiempo EMG(s)", "Amplitud(V)", "Tiempo DPT(s)", "Distancia (cm)", "Potencia optica derecho", "Potencia optica izquierdo"]) -> ()  [unwired: 1 in]
                                }
                              }
                            }
                            frame #2 {
                              # "Si el usuario desea repetir el experimento se vuelve al estado inicio en donde se espera que comience el experimento. De lo contrario se sale del loop y vuelve al menu principal."
                              n457 = Two Button Dialog(message="¿Desea repetir el experimento?", 1:"No" ("F button name (\"Cancel\")"), 2:"Si" ("T button name (\"OK\")")) -> (T button?=w909:bool)
                              n458 = Not(x=w909) -> (.not. x?=→"T button?":bool)
                            }
                          }
                        }
                      }
                      n459 = local read "T button?"() -> (w540:bool)
                    }
                  }
                }
                "Array 2" <- w448
              }
            }
          }
          event Timeout {
            n460 = event-data() -> ()  [unwired: 1 in, 3 out]
          }
        }
        "Array 3" <- w31
      }
      "Array 4" <- w22
    }
  }
